vi "Do_ADAM_channel.vi"(4 "Scan Period":dbl format="%.2f", 5 "Previous Scan Value":dbl format="%.2f", 6 "Present scan array":dbl[](array[numeric]) format="%.2f", 7 "Value to Output":dbl format="%.2f", 8 "Ch Description":T1 {"Duty" format="%.0b"; "D" format="%#_5g"; "C" format="%#_5g"; "B" format="%#_5g"; "A" format="%#_5g"}, 9 "Ch names":string[](array[string])) -> (0 "Scan comment":string, 1 "Output":dbl format="%.3f")   [LabVIEW 2015]
uses:
  ADAM Client/Sub VIs/ADAM Controls/Ch_description_ADAM.ctl
  ADAM Client/Sub VIs/ADAM Controls/Module_type_ADAM.ctl
  ADAM Client/Sub VIs/ADAM Controls/Function_ADAM.ctl
  ADAM Client/Sub VIs/ADAM Controls/Channel_State.ctl
  ADAM Client/Sub VIs/ADAM Controls/Calib_type_ADAM.ctl
  ADAM Client/Sub VIs/ADAM Controls/Address.ctl
  ADAM Client/Sub VIs/ADAM Controls/Remember_value_mode.ctl
  ADAM Serial/Instrument drivers/Arduino/ctls_and_globals/Arduino tx msg cluster.ctl
  ADAM Client/Sub VIs/ADAM Controls/Search_mode.ctl
  Anemometry/Anemometry Sub Vis/Controls/In_Range.ctl
  <vilib>/Analysis/baseanly.llb/Mean (DBL).vi
  ADAM_Global.vi
  Anemometry/Anemometry Sub Vis/Globals/Gas_management_global.vi
  Anemometry/Anemometry Sub Vis/Globals/Constants_global.vi
  <vilib>/Analysis/NI_AALBase.lvlib
panel:
  in  "History Length":i32=150
  in  "K_Uni_chilled water":dbl=4.5
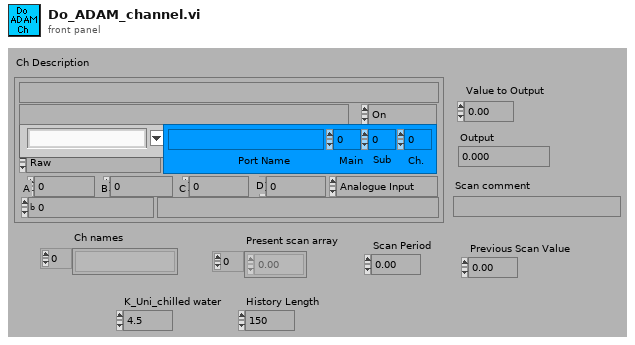
[diagram p1: front panel]
types:
  T1 = typedef "Ch_description_ADAM.ctl" = cluster{"Ch Name":string, "Type":T2, "Function":T3, "Ch State":T4, "Calibration type":T5, "A":dbl, "B":dbl, "C":dbl, "D":dbl, "Comments":string, "Address":T6, "String":string, "Duty":u16}
  T2 = typedef "Module_type_ADAM.ctl" = string
  T3 = typedef "Function_ADAM.ctl" = enum16{"Analogue Input", "Digital Input", "Event counter", "Event rate", "Analogue Output", "Digital Output", "Relay Output"}
  T4 = typedef "Channel_State.ctl" = enum16{"On", "Off", "Always On", "Always Off"}
  T5 = typedef "Calib_type_ADAM.ctl" = enum16{"Raw", "Bx + A", "Cx^2 + Bx + A", "Dx^3 + Cx^2 + Bx + A", "In Band", "Hi-Tec Q", "Hi-Tec M_dot", "Text"}
  T6 = typedef "Address.ctl" = cluster{"Main":i32, "Ch.":i32, "Sub":i32, "Port Name":string}
  T7 = typedef "Remember_value_mode.ctl" = enum16{"Read only", "Read and Write"}
  T8 = typedef "Search_mode.ctl" = enum16{"Between times", "All Times"}
  T9 = typedef "In_Range.ctl" = enum16{"%", "±", "% & ±"}
  T10 = typedef "Arduino tx msg cluster.ctl" = cluster{"dest":u8, "A/D/C/I":string, "R/W":string, "chan":u8, "val (float)":sgl}
  T11 = typedef "Client_State_Cluster.ctl" = cluster{"Client Name":string, "Traverse level State":T12, "People to Email":string[], "Next Contact Time":dbl}
  T12 = typedef "Traverse_Level_State.ctl" = enum16{"Running", "Complete"}
  T13 = cluster{"Centre Times":dbl[], "Output array":dbl[]}
  T14 = cluster{"Centre Times":dbl[], "Output array":dbl[]}[]
  T15 = typedef "Valco_valve_ph.ctl" = u16
  T16 = typedef "LVDateTimeRec.ctl" = cluster{"fractional second":dbl, "second":i32, "minute":i32, "hour":i32, "day of month":i32, "month":i32, "year":i32, "day of week":i32, "day of year":i32, "DST":i32}
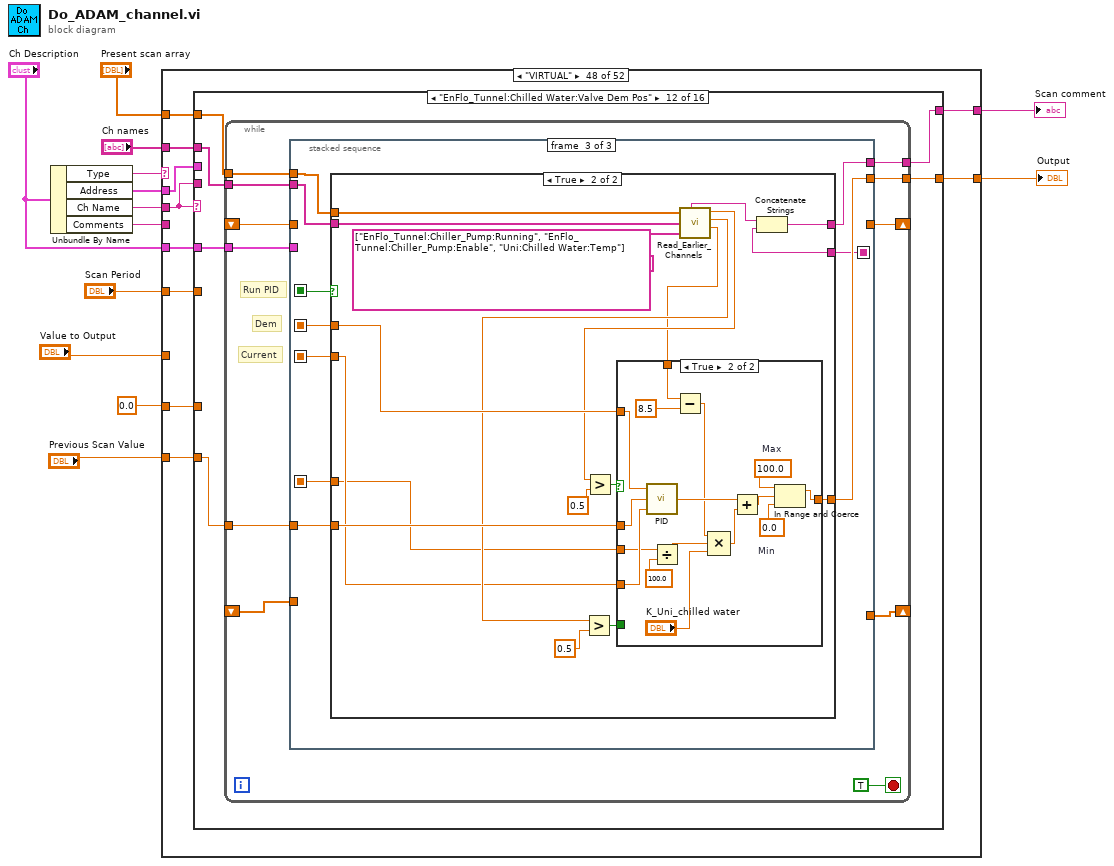
[diagram p0: block diagram]
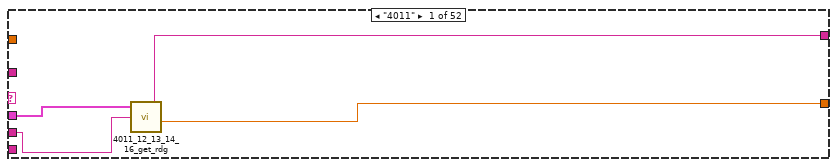
[diagram p2: hidden frame]
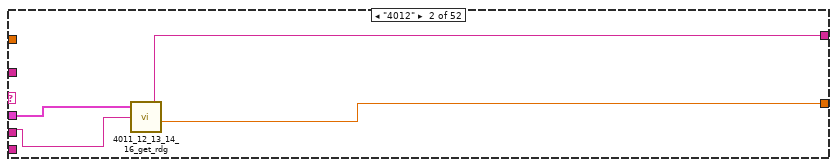
[diagram p3: hidden frame]
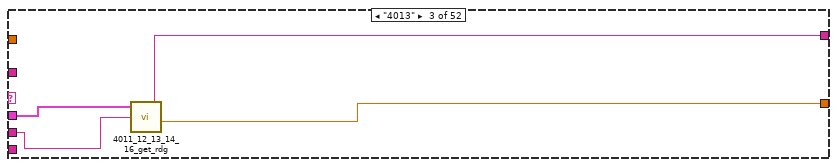
[diagram p4: hidden frame]
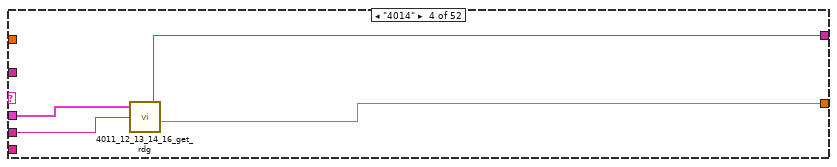
[diagram p5: hidden frame]
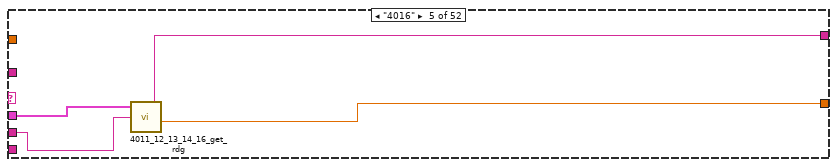
[diagram p6: hidden frame]
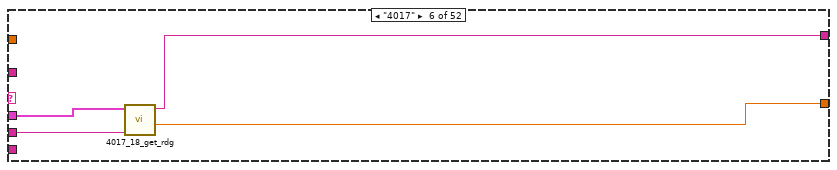
[diagram p7: hidden frame]
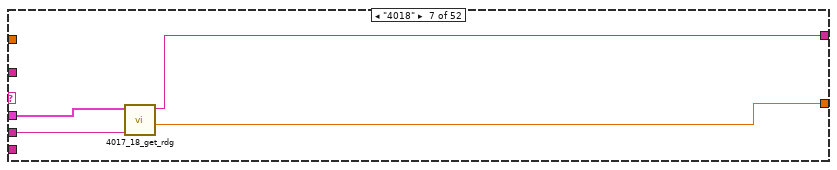
[diagram p8: hidden frame]
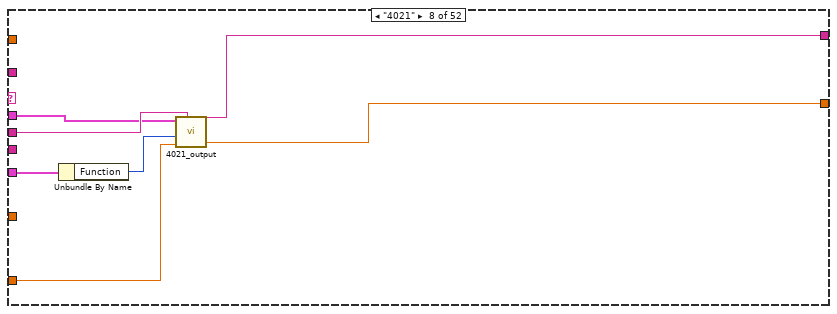
[diagram p9: hidden frame]
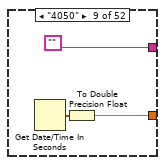
[diagram p10: hidden frame]
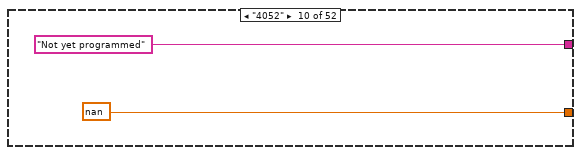
[diagram p11: hidden frame]
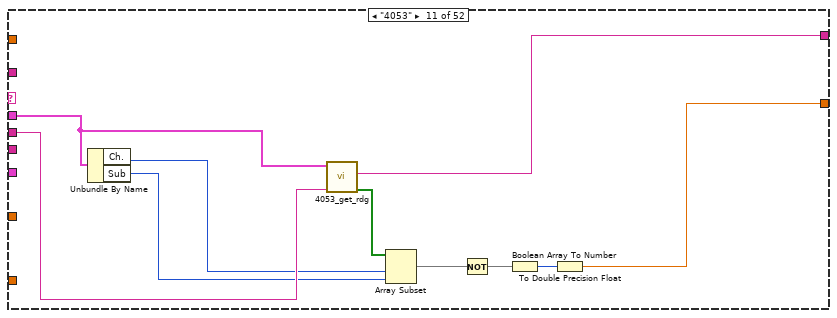
[diagram p12: hidden frame]
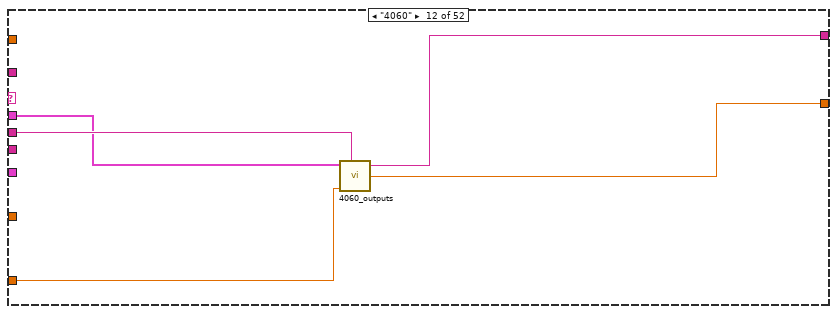
[diagram p13: hidden frame]
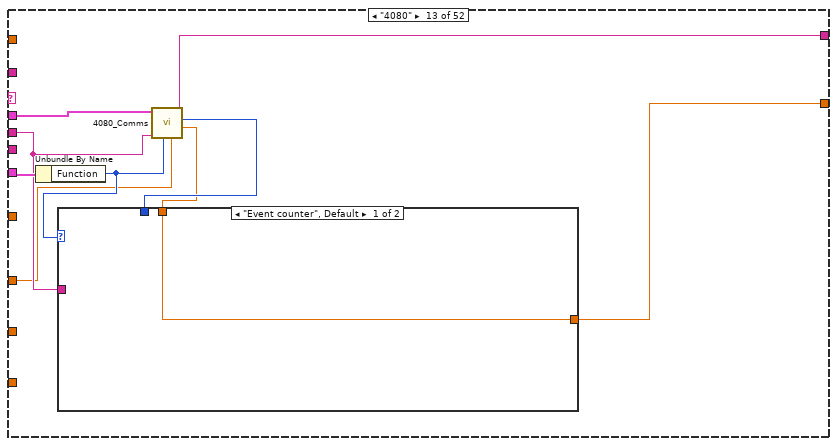
[diagram p14: hidden frame]
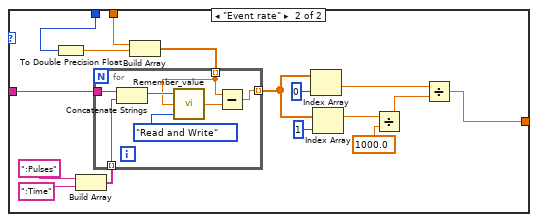
[diagram p15: hidden frame]
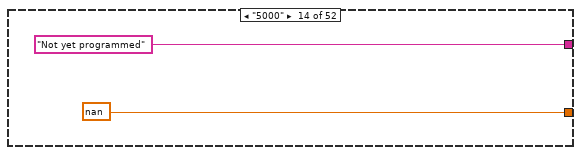
[diagram p16: hidden frame]
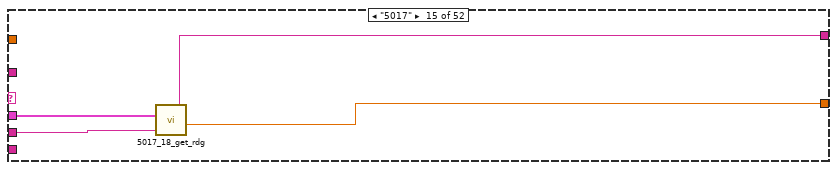
[diagram p17: hidden frame]
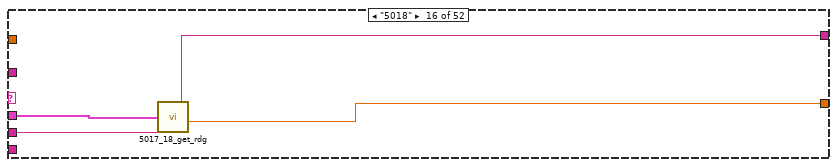
[diagram p18: hidden frame]
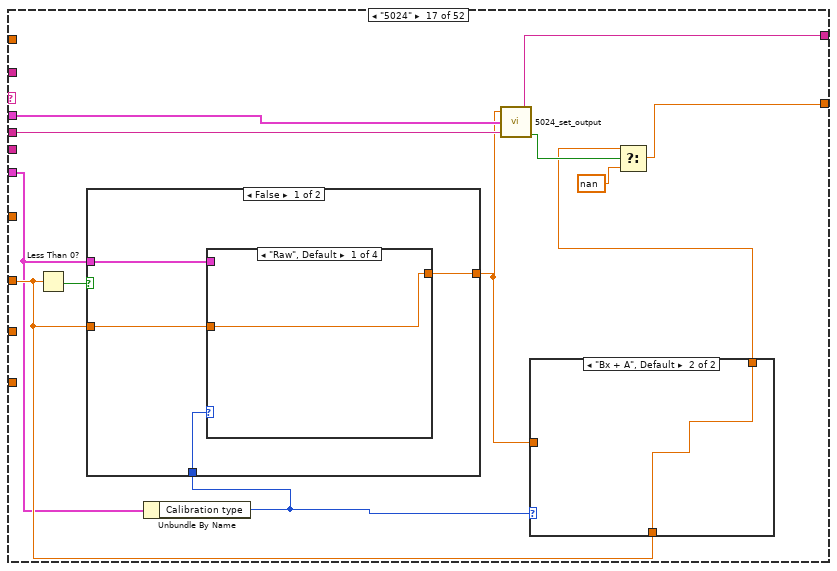
[diagram p19: hidden frame]
diagram:
  n1 = Unbundle By Name("Ch Description") -> ("Type"=w11:T2, "Address"=w10:T6, "Ch Name"=w2:string, "Comments"=w7:string)
  n2 = case shown="\"VIRTUAL\"" w11 {
    tunnel: [w16 w20 w24 w28 w32 w36 w40 w47 w50 nan w57 w66 w75 nan w105 w109 w119 w151 w159 w180 w202 w221 w236 w252 w281 w301 w389 w402 w404 w406 nan w514 w515 w518 w534 w546 0.0 ("Output") w555 w556 w560 w568 w599 w607 w690 w691 w697 w771 w819 w1340 nan w1371 w1397] -> w8
    tunnel: [w17 w21 w25 w29 w33 w37 w41 w48 "" "Not yet programmed" w62 w67 w77 "Not yet programmed" w106 w110 w122 w152 w158 w181 w203 w220 w239 w254 w276 w298 "" w403 "" w427 "Not yet programmed" w513 "" w519 w533 w547 "Warning; unmatched case in Do_ADAM_channel" ("Status note") w554 "" w561 w567 w598 w601 "Crazy time based random number!" w695 w699 w763 w818 w1341 "Not yet programmed" w1360 ""] -> w5
    tunnel: w10 -> [w14 w18 w22 w26 w30 w34 w38 w42 _ _ w54 w65 w69 _ w107 w111 w123 w153 w157 w182 w204 w235 w251 w267 w292 _ _ w401 _ _ _ w511 _ w517 w536 w549 _ w552 _ _ _ _ _ _ w693 w701 w768 w810 w1346 _ _ w1406]
    tunnel: "Ch Description" -> [_ _ _ _ _ _ _ w46 _ _ _ _ w76 _ _ _ w112 _ w156 w179 w201 _ _ _ _ w305 _ _ _ w432 _ _ _ _ _ _ _ _ w557 w562 w573 w600 w605 _ _ w700 _ w812 _ _ _ _]
    tunnel: w2 -> [w15 w19 w23 w27 w31 w35 w39 w43 _ _ w63 w68 w72 _ w104 w108 w118 w150 w154 w176 w198 _ _ _ _ _ w385 _ _ _ _ w512 _ _ w535 w548 _ w553 _ _ _ _ _ _ w694 w698 w764 w815 w1345 _ w1367 _]
    tunnel: "Ch names" -> [_ _ _ _ _ _ _ _ _ _ _ _ _ _ _ _ _ _ _ _ _ _ _ _ _ w310 _ _ _ w431 _ _ _ _ _ _ _ _ _ w563 w574 _ w613 _ _ _ _ w817 _ _ _ _]
    tunnel: "Present scan array" -> [_ _ _ _ _ _ _ _ _ _ _ _ _ _ _ _ _ _ _ _ _ _ _ _ _ w309 _ _ _ w429 _ _ _ _ _ _ _ _ _ w564 w571 _ w612 _ _ _ _ w816 _ _ _ _]
    tunnel: w7 -> [_ _ _ _ _ _ _ _ _ _ _ _ _ _ _ _ _ _ _ _ _ _ _ _ _ w308 _ _ _ w433 _ _ _ _ _ _ _ _ _ _ w566 _ w611 _ _ _ _ _ _ _ _ _]
    tunnel: "Value to Output" -> [_ _ _ _ _ _ _ w44 _ _ _ w64 w70 _ _ _ w114 _ w155 w177 w199 _ w237 w253 _ _ _ _ _ _ _ _ _ _ w532 _ _ _ _ _ w572 _ _ _ _ w696 w772 _ _ _ _ w1401]
    tunnel: "Scan Period" -> [_ _ _ _ _ _ _ _ _ _ _ _ _ _ _ _ _ _ _ _ _ _ _ _ _ w300 _ _ _ _ _ _ _ _ _ _ _ _ _ _ w569 _ w606 _ _ _ _ w814 _ _ _ _]
    tunnel: "Previous Scan Value" -> [_ _ _ _ _ _ _ _ _ _ _ _ _ _ _ _ _ _ _ _ _ w223 _ _ w268 _ _ _ w404 w407 _ _ w515 _ _ _ _ _ _ _ w570 _ _ _ _ _ _ w813 _ _ _ _]
    tunnel: 0.0 -> [_ _ _ _ _ _ _ _ _ _ _ _ _ _ _ _ _ _ _ _ _ _ _ _ _ _ _ _ _ _ _ _ _ _ _ _ _ _ _ _ _ _ _ _ _ _ _ w811 _ _ _ _]
    frame "4011" {
      n3 = call "4011_12_13_14_16_get_rdg.vi"("Address"=w14, "Channel Name"=w15) -> ("Comment"=w17:string, "Reading"=w16:dbl)  [unwired: 1 in, 2 out]
    }
    frame "4012" {
      n4 = call "4011_12_13_14_16_get_rdg.vi"("Address"=w18, "Channel Name"=w19) -> ("Comment"=w21:string, "Reading"=w20:dbl)  [unwired: 1 in, 2 out]
    }
    frame "4013" {
      n5 = call "4011_12_13_14_16_get_rdg.vi"("Address"=w22, "Channel Name"=w23) -> ("Comment"=w25:string, "Reading"=w24:dbl)  [unwired: 1 in, 2 out]
    }
    frame "4014" {
      n6 = call "4011_12_13_14_16_get_rdg.vi"("Address"=w26, "Channel Name"=w27) -> ("Comment"=w29:string, "Reading"=w28:dbl)  [unwired: 1 in, 2 out]
    }
    frame "4016" {
      n7 = call "4011_12_13_14_16_get_rdg.vi"("Address"=w30, "Channel Name"=w31) -> ("Comment"=w33:string, "Reading"=w32:dbl)  [unwired: 1 in, 2 out]
    }
    frame "4017" {
      n8 = call "4017_18_get_rdg.vi"("Channel Name"=w35, "Address"=w34) -> ("Reading"=w36:dbl, "Comment"=w37:string)  [unwired: 2 in, 2 out]
    }
    frame "4018" {
      n9 = call "4017_18_get_rdg.vi"("Channel Name"=w39, "Address"=w38) -> ("Reading"=w40:dbl, "Comment"=w41:string)  [unwired: 2 in, 2 out]
    }
    frame "4021" {
      n10 = Unbundle By Name(w46) -> ("Function"=w45:T3)
      n11 = call "4021_output.vi"("Address"=w42, "Function"=w45, "Set to:"=w44, "Channel Name"=w43) -> ("Comment"=w48:string, "Reading"=w47:dbl)  [unwired: 1 in, 1 out]
    }
    frame "4050" {
      n12 = Get Date/Time In Seconds() -> (seconds since 1Jan1904=w49:timestamp)
      n13 = To Double Precision Float(number=w49) -> (double precision float=w50:dbl)
    }
    frame "4052" {
    }
    frame "4053" {
      n14 = Unbundle By Name(w54) -> ("Ch."=w55:i32, "Sub"=w61:i32)
      n15 = call "4053_get_rdg.vi"("Channel Name"=w63, "Address"=w54) -> ("Boolean array"=w60:bool[], "Comment"=w62:string)  [unwired: 2 in, 2 out]
      n16 = Array Subset(array=w60, index=w55, length=w61) -> (w59:bool[])
      n17 = Not(x=w59) -> (.not. x?=w56:bool[])
      n18 = Boolean Array To Number(Boolean array=w56) -> (number=w58:u32)
      n19 = To Double Precision Float(number=w58) -> (double precision float=w57:dbl)
    }
    frame "4060" {
      n20 = call "4060_outputs.vi"("Address"=w65, "Value to Output"=w64, "Channel Name"=w68) -> ("Comment"=w67:string, "Reading"=w66:dbl)  [unwired: 2 in, 1 out]
    }
    frame "4080" {
      n21 = Unbundle By Name(w76) -> ("Function"=w71:T3)
      n22 = call "4080_Comms.vi"("Value to display"=w70, "Function"=w71, "Channel Name"=w72, "Address"=w69) -> ("Reading"=w73:dbl, "millisecond timer value"=w74:u32, "Comment"=w77:string)  [unwired: 2 in, 1 out]
      n23 = case shown="\"Event counter\", Default" w71 {
        tunnel: w72 -> [_ w94]
        tunnel: w74 -> [_ w87]
        tunnel: [w78 w79] -> w75
        tunnel: w73 -> [w78 w88]
        frame "Event counter", Default {
        }
        frame "Event rate" {
          n24 = To Double Precision Float(number=w87) -> (double precision float=w86:dbl)
          n25 = Build Array(":Pulses", ":Time") -> (w89:string[])
          n26 = Build Array(w88, w86) -> (w85:dbl[])
          n27 = for {
            tunnel: w94 -> [w98]
            tunnel: [w99] -> w82 mode=indexing
            tunnel: w89 -> [w96] mode=indexing
            tunnel: w85 -> [w95] mode=indexing
            n28 = Concatenate Strings(w98, w96) -> (w97:string)
            n29 = call "Remember_value.vi"("Mode"=Remember_value_mode."Read and Write", "Input Value"=w95, "Ch name"=w97) -> ("Output Value"=w100:dbl)
            n30 = Subtract(x=w95, y=w100) -> (x-y=w99:dbl)
          }
          n31 = Index Array(array=w82, index=0) -> (element=w80:dbl)
          n32 = Index Array(array=w82, index=1) -> (element=w81:dbl)
          n33 = Divide(x=w81, y=1000.0) -> (x/y=w92:dbl)
          n34 = Divide(x=w80, y=w92) -> (x/y=w79:dbl)
        }
      }
    }
    frame "5000" {
    }
    frame "5017" {
      n35 = call "5017_18_get_rdg.vi"("Address (all reqd.)"=w107, "Channel Name"=w104) -> ("Comment"=w106:string, "Reading"=w105:dbl)  [unwired: 3 out]
    }
    frame "5018" {
      n36 = call "5017_18_get_rdg.vi"("Address (all reqd.)"=w111, "Channel Name"=w108) -> ("Comment"=w110:string, "Reading"=w109:dbl)  [unwired: 3 out]
    }
    frame "5024" {
      n37 = Less Than 0?(x=w114) -> (x < 0?=w117:bool)
      n38 = Unbundle By Name(w112) -> ("Calibration type"=w113:T5)
      n39 = case shown="False" w117 {
        tunnel: [w129 0.0 ("t")] -> w115
        tunnel: w114 -> [w127 _]
        tunnel: w113 -> [w128 _]
        tunnel: w112 -> [w126 _]
        frame False {
          n40 = case shown="\"Raw\", Default" w128 {
            tunnel: w127 -> [w130 w133 w139 w145]
            tunnel: w126 -> [_ w136 w142 w148]
            tunnel: [w130 w131 w137 w143] -> w129
            frame "Raw", Default {
            }
            frame "Bx + A" {
              n41 = Unbundle By Name(w136) -> ("A"=w135:dbl)
              n42 = Equal?(x=w135, y=w133) -> (x = y?=w134:bool)
              n43 = Select(t=0.0, s=w134, f=w133) -> (s? t:f=w131:dbl)
            }
            frame "Cx^2 + Bx + A" {
              n44 = Unbundle By Name(w142) -> ("A"=w141:dbl)
              n45 = Equal?(x=w141, y=w139) -> (x = y?=w140:bool)
              n46 = Select(t=0.0, s=w140, f=w139) -> (s? t:f=w137:dbl)
            }
            frame "Dx^3 + Cx^2 + Bx + A" {
              n47 = Unbundle By Name(w148) -> ("A"=w147:dbl)
              n48 = Equal?(x=w147, y=w145) -> (x = y?=w146:bool)
              n49 = Select(t=0.0, s=w146, f=w145) -> (s? t:f=w143:dbl)
            }
          }
        }
        frame True {
        }
      }
      n50 = call "5024_set_output.vi"("Set to:"=w115, "Address (all reqd.)"=w123, "Channel Name"=w118) -> ("Comment"=w122:string, "Good Reply"=w120:bool)  [unwired: 2 out]
      n51 = case shown="\"Bx + A\", Default" w113 {
        tunnel: [w124 w125] -> w116
        tunnel: w115 -> [w124 _]
        tunnel: w114 -> [_ w125]
        frame "Raw" {
        }
        frame "Bx + A", Default {
        }
      }
      n52 = Select(t=w116, s=w120, f=nan) -> (s? t:f=w119:dbl)
    }
    frame "5051" {
      n53 = call "5051_56_get_inputs.vi"("Address (Main, Sub reqd.)"=w153, "Channel Name"=w150) -> ("Comment"=w152:string, "Single output"=w151:dbl)  [unwired: 3 out]
    }
    frame "5056" {
      n54 = Unbundle By Name(w156) -> ("Function"=w160:T3)
      n55 = case shown="\"Digital Input\"" w160 {
        tunnel: w157 -> [_ w166 w175]
        tunnel: ["This function is not available" w167 w173] -> w158
        tunnel: [nan ("A") w164 w170] -> w159
        tunnel: w155 -> [_ _ w169]
        tunnel: w154 -> [_ w163 w168]
        frame "Analogue Input", Default {
        }
        frame "Digital Input" {
          # "Readback value"
          n56 = call "5060_check_outputs.vi"("Address (Main, Sub reqd.)"=w166, "Channel Name"=w163) -> ("Comment"=w167:string, "Single Channel"=w165:i16)  [unwired: 3 out]
          n57 = To Double Precision Float(number=w165) -> (double precision float=w164:dbl)
        }
        frame "Relay Output" {
          # "Sets single o/p channel"
          n58 = Greater Than 0?(x=w169) -> (x > 0?=w174:bool)
          n59 = call "5056_60_set_single_output.vi"("Channel Name"=w168, "Address (all reqd.)"=w175, "Set state:"=w174) -> ("Comment"=w173:string, "Good Reply"=w172:bool)  [unwired: 2 out]
          n60 = Select(t=w169, s=w172, f=nan) -> (s? t:f=w170:dbl)
        }
      }
    }
    frame "5060" {
      n61 = Unbundle By Name(w179) -> ("Function"=w178:T3)
      n62 = case shown="\"Relay Output\"" w178 {
        tunnel: w182 -> [_ w188 w197]
        tunnel: ["This function is not available" w189 w195] -> w181
        tunnel: [nan ("A") w186 w192] -> w180
        tunnel: w177 -> [_ _ w191]
        tunnel: w176 -> [_ w185 w190]
        frame "Analogue Input", Default {
        }
        frame "Digital Input" {
          # "Readback value"
          n63 = call "5060_check_outputs.vi"("Address (Main, Sub reqd.)"=w188, "Channel Name"=w185) -> ("Comment"=w189:string, "Single Channel"=w187:i16)  [unwired: 3 out]
          n64 = To Double Precision Float(number=w187) -> (double precision float=w186:dbl)
        }
        frame "Relay Output" {
          # "Sets single o/p channel"
          n65 = Greater Than 0?(x=w191) -> (x > 0?=w196:bool)
          n66 = call "5056_60_set_single_output.vi"("Channel Name"=w190, "Address (all reqd.)"=w197, "Set state:"=w196) -> ("Comment"=w195:string, "Good Reply"=w194:bool)  [unwired: 2 out]
          n67 = Select(t=w191, s=w194, f=nan) -> (s? t:f=w192:dbl)
        }
      }
    }
    frame "6060" {
      n68 = Unbundle By Name(w201) -> ("Function"=w200:T3)
      n69 = case shown="\"Digital Input\"" w200 {
        tunnel: w204 -> [_ w210 w219]
        tunnel: ["This function is not available" w211 w217] -> w203
        tunnel: [nan ("A") w208 w214] -> w202
        tunnel: w199 -> [_ _ w213]
        tunnel: w198 -> [_ w207 w212]
        frame "Analogue Input", Default {
        }
        frame "Digital Input" {
          n70 = call "6060_read_all_I-O.vi"("Address (Main, Sub reqd.)"=w210, "Channel Name"=w207) -> ("Comment"=w211:string, "Single Input Channel"=w209:i16)  [unwired: 3 out]
          n71 = To Double Precision Float(number=w209) -> (double precision float=w208:dbl)
        }
        frame "Relay Output" {
          # "Sets single o/p channel"
          n72 = Greater Than 0?(x=w213) -> (x > 0?=w218:bool)
          n73 = call "6060_set_single_output.vi"("Channel Name"=w212, "Address (Main, Ch requd.)"=w219, "Set state:"=w218) -> ("Comment"=w217:string, "Good Reply"=w216:bool)  [unwired: 2 out]
          n74 = Select(t=w213, s=w216, f=nan) -> (s? t:f=w214:dbl)
        }
      }
    }
    frame "Arduino A_in" {
      w229 = T10 {"dest"=1, "A/D/C/I"="A", "R/W"="R", "chan"=1, "val (float)"=0.0}  # Tx msg cluster
      # "Analogue read case"
      n75 = Unbundle By Name(w235) -> ("Port Name"=w226:string, "Main"=w227:i32, "Ch."=w228:i32)
      n76 = To Unsigned Byte Integer(number=w227) -> (unsigned 8bit integer=w234:u8)
      n77 = To Unsigned Byte Integer(number=w228) -> (unsigned 8bit integer=w232:u8)
      n78 = Bundle By Name(cluster=w229, "dest"=w234, "A/D/C/I"="A" ("A/D"), "R/W"="R", "chan"=w232, "val (float)"=sgl 0.0) -> (w225:T10)
      n79 = call "Arduino generic wrapper.vi"("Tx msg cluster"=w225, "Port name"=w226) -> ("Scan comment"=w220:string, "Output"=w222:dbl)
      n80 = Empty String/Path?(string/path=w220) -> (empty?=w224:bool)
      n81 = Select(t=w222, s=w224, f=w223) -> (s? t:f=w221:dbl)
    }
    frame "Arduino A_out" {
      w246 = T10 {"dest"=1, "A/D/C/I"="A", "R/W"="R", "chan"=1, "val (float)"=0.0}  # Tx msg cluster
      # "Analogue write case"
      n82 = Unbundle By Name(w251) -> ("Port Name"=w243:string, "Main"=w244:i32, "Ch."=w245:i32)
      n83 = To Unsigned Byte Integer(number=w244) -> (unsigned 8bit integer=w250:u8)
      n84 = To Unsigned Byte Integer(number=w245) -> (unsigned 8bit integer=w249:u8)
      n85 = To Single Precision Float(number=w237) -> (single precision float=w241:sgl)
      n86 = Bundle By Name(cluster=w246, "dest"=w250, "A/D/C/I"="A" ("A/D"), "R/W"="W", "chan"=w249, "val (float)"=w241) -> (w242:T10)
      n87 = call "Arduino generic wrapper.vi"("Tx msg cluster"=w242, "Port name"=w243) -> ("Scan comment"=w239:string)  [unwired: 1 out]
      n88 = Empty String/Path?(string/path=w239) -> (empty?=w238:bool)
      n89 = Select(t=w237, s=w238, f=nan ("Reading")) -> (s? t:f=w236:dbl)
    }
    frame "Arduino D_out" {
      w262 = T10 {"dest"=1, "A/D/C/I"="A", "R/W"="R", "chan"=1, "val (float)"=0.0}  # Tx msg cluster
      # "Digital write case"
      n90 = Unbundle By Name(w267) -> ("Port Name"=w259:string, "Main"=w260:i32, "Ch."=w261:i32)
      n91 = To Unsigned Byte Integer(number=w260) -> (unsigned 8bit integer=w266:u8)
      n92 = To Unsigned Byte Integer(number=w261) -> (unsigned 8bit integer=w265:u8)
      n93 = To Single Precision Float(number=w253) -> (single precision float=w257:sgl)
      n94 = Bundle By Name(cluster=w262, "dest"=w266, "A/D/C/I"="D" ("A/D"), "R/W"="W", "chan"=w265, "val (float)"=w257) -> (w258:T10)
      n95 = call "Arduino generic wrapper.vi"("Tx msg cluster"=w258, "Port name"=w259) -> ("Scan comment"=w254:string)  [unwired: 1 out]
      n96 = Empty String/Path?(string/path=w254) -> (empty?=w255:bool)
      n97 = Select(t=w253, s=w255, f=nan ("Reading")) -> (s? t:f=w252:dbl)
    }
    frame "Arduino Thermistor" {
      w286 = T10 {"dest"=1, "A/D/C/I"="A", "R/W"="R", "chan"=1, "val (float)"=0.0}  # Tx msg cluster
      # "Thermistor read case"
      # "values not expected in 'normal' operating conditions"
      n98 = Unbundle By Name(w292) -> ("Port Name"=w283:string, "Main"=w284:i32, "Ch."=w285:i32)
      n99 = To Unsigned Byte Integer(number=w284) -> (unsigned 8bit integer=w291:u8)
      n100 = To Unsigned Byte Integer(number=w285) -> (unsigned 8bit integer=w289:u8)
      n101 = Bundle By Name(cluster=w286, "dest"=w291, "A/D/C/I"="A" ("A/D"), "R/W"="R", "chan"=w289, "val (float)"=sgl 0.0) -> (w282:T10)
      n102 = call "Arduino generic wrapper.vi"("Tx msg cluster"=w282, "Port name"=w283) -> ("Scan comment"=w272:string, "Output"=w270:dbl)
      n103 = Empty String/Path?(string/path=w272) -> (empty?=w271:bool)
      n104 = Select(t=w270, s=w271, f=w268) -> (s? t:f=w269:dbl)
      n105 = Less?(x=w270, y=-40.0) -> (x < y?=w273:bool)
      n106 = Greater?(x=w270, y=140.0) -> (0:w274:bool)
      n107 = case shown="False" w273 {
        tunnel: [w294 "Faulty thermistor open-circuit;"] -> w275
        tunnel: w274 -> [w293 _]
        frame False {
          n108 = case shown="True" w293 {
            tunnel: ["" "Faulty thermistor short-circuit;"] -> w294
            frame False {
            }
            frame True {
            }
          }
        }
        frame True {
        }
      }
      n109 = Or(x=w273, y=w274) -> (x .or. y?=w278:bool)
      n110 = Select(t=nan ("f"), s=w278, f=w269) -> (s? t:f=w281:dbl)
      n111 = Concatenate Strings(w272, w275) -> (w276:string)
    }
    frame "Average" {
      # "The Channel names to average must appear in the comments field separated by semi colons"
      n112 = call "Get_array_values_fr_String.vi"("String Value"=w308) -> ("String array"=w307:string[])  [unwired: 1 out]
      n113 = Equal To 0?(x=w300) -> (x = 0?=w299:bool)
      n114 = global read "ADAM_Global.vi" "Active Ch names"() -> (w306:string[])
      n115 = case shown="False" w299 {
        tunnel: w305 -> [w314 _]
        tunnel: [w312 TRUE] -> w304
        tunnel: [w311 2.0 ("A")] -> w303
        frame False {
          n116 = Unbundle By Name(w314) -> ("D"=w311:dbl)
          n117 = Less?(x=w311, y=2.0) -> (x < y?=w312:bool)
        }
        frame True {
        }
      }
      n118 = case shown="True" w304 {
        tunnel: w310 -> [_ w349]
        tunnel: w309 -> [_ w348]
        tunnel: w307 -> [w319 w347]
        tunnel: [w317 w345] -> w298
        tunnel: w306 -> [_ w344]
        tunnel: [w320 w343] -> w302
        tunnel: w303 -> [w321 _]
        frame False {
          w328 = FALSE  # All Active Channels
          n119 = Get Date/Time In Seconds() -> (seconds since 1Jan1904=w331:timestamp)
          n120 = To Double Precision Float(number=w331) -> (double precision float=w329:dbl)
          n121 = Subtract(x=w329, y=w321) -> (x-y=w330:dbl)
          n122 = call "Get_ADAM_averages_server.vi"("No of averages"=1, "All Active Channels"=w328, "End time"=w329, "Start time"=w330, "Clients time"=w329, "ADAM Ch Names"=w319) -> ("DBL values"=w326:dbl[][])  [unwired: 4 out]
          n123 = Index Array(array=w326, index (row)=0) -> (element=w323:dbl[])  [unwired: 1 in]
          n124 = Array Subset(array=w323, index=1) -> (w322:dbl[])  [unwired: 1 in]
          n125 = for {
            tunnel: w322 -> [w337] mode=indexing
            tunnel: [w337] -> w320 mode=indexing if=w335
            tunnel: w319 -> [w334] mode=indexing
            shift-right: [w332] -> w317
            shift-left: "" -> [w333]
            n126 = Not A Number/Path/Refnum?(number/path/refnum=w337) -> (NaN/Path/Refnum?=w336:bool)
            n127 = Not(x=w336) -> (.not. x?=w335:bool)
            n128 = case shown="False" w335 {
              tunnel: w334 -> [w340 _]
              tunnel: w333 -> [w339 w342]
              tunnel: [w338 w342] -> w332
              frame False {
                n129 = Format Into String(format string="Channel \"%s\" is not currently active.\n", initial string=w339, w340) -> (resulting string=w338:string)  [unwired: 1 in, 1 out]
              }
              frame True {
              }
            }
          }
        }
        frame True {
          n130 = for {
            tunnel: w349 -> [w362]
            tunnel: w348 -> [w361]
            tunnel: w347 -> [w358] mode=indexing
            shift-right: [w359] -> w345
            shift-left: "" -> [w360]
            tunnel: [w352] -> w343 mode=indexing if=w350
            tunnel: w344 -> [w353]
            n131 = call "Read_value_of_earlier_Ch.vi"("Desired Ch to Read"=w358, "Ch names"=w362, "Present scan array"=w361) -> ("Value"=w356:dbl, "Scan comment"=w355:string)  [unwired: 1 in]
            n132 = Not A Number/Path/Refnum?(number/path/refnum=w356) -> (NaN/Path/Refnum?=w357:bool)
            n133 = case shown="False" w357 {
              tunnel: w358 -> [w365 _]
              tunnel: [w368 w378] -> w352
              tunnel: w356 -> [w367 w378]
              tunnel: [w370 w377] -> w354
              tunnel: w355 -> [w369 w377]
              tunnel: w353 -> [w366 _]
              frame False {
                n134 = Search 1D Array(1D array=w366, element=w365) -> (index of element=w363:i32)  [unwired: 1 in]
                n135 = Greater Or Equal To 0?(x=w363) -> (x >= 0?=w364:bool)
                n136 = case shown="False" w364 {
                  tunnel: w365 -> [w374 _]
                  tunnel: [w373 w376] -> w370
                  tunnel: w369 -> [_ w376]
                  tunnel: [nan w375] -> w368
                  tunnel: w367 -> [_ w375]
                  frame False {
                    n137 = Format Into String(format string="Channel \"%s\" is not currently active.\n", w374) -> (resulting string=w373:string)  [unwired: 2 in, 1 out]
                  }
                  frame True {
                  }
                }
              }
              frame True {
              }
            }
            n138 = Concatenate Strings(w360, w354) -> (w359:string)
            n139 = Not A Number/Path/Refnum?(number/path/refnum=w352) -> (NaN/Path/Refnum?=w351:bool)
            n140 = Not(x=w351) -> (.not. x?=w350:bool)
          }
        }
      }
      n141 = call-poly <vilib>:"Mean.vi"("X"=w302) -> ("mean"=w301:dbl)  [unwired: 1 out]
    }
    frame "Client Info" {
      n142 = global read "ADAM_Global.vi" "Client State Array"() -> (w391:T11[])
      n143 = call "Split_Ch_name.vi"("Ch name"=w385) -> ("Top level"=w383:string, "Low level"=w381:string)  [unwired: 1 out]
      n144 = Equal?(x="Status" ("Substring"), y=w383) -> (x = y?=w382:bool)
      n145 = Select(t=w381, s=w382, f="") -> (s? t:f=w379:string)
      n146 = for {
        tunnel: w391 -> [w400] mode=indexing
        tunnel: [w399] -> w392 mode=indexing
        n147 = Unbundle By Name(w400) -> ("Client Name"=w399:string)
      }
      n148 = Search 1D Array(1D array=w392, element=w379) -> (index of element=w387:i32)  [unwired: 1 out]
      n149 = Less Than 0?(x=w387) -> (x < 0?=w386:bool)
      n150 = Index Array(array=w391, index=w387) -> (element=w390:T11)
      n151 = case shown="False" w386 {
        tunnel: w390 -> [w395 _]
        tunnel: w379 -> [w394 w397]
        tunnel: [w393 w396] -> w389
        frame False {
          n152 = call "Get_Client_Status_string.vi"("Client State Cluster"=w395, "Client Name"=w394) -> ("Code Value"=w393:dbl)  [unwired: 1 in]
        }
        frame True {
          w396 = 7.0 ("Code Value")
          n153 = call "Remember_value.vi"("Mode"=Remember_value_mode."Read and Write", "Input Value"=w396, "Ch name"=w397) -> ()  [unwired: 1 out]
        }
      }
    }
    frame "ClimatronicsUDP" {
      n154 = call "ClimatronicsUDP_get_rdg.vi"("Address"=w401) -> ("Output"=w402:dbl, "Status note"=w403:string)  [unwired: 5 in]
    }
    frame "Coded" {
    }
    frame "Comparator" {
      # "A Warn if above this value\nB Warn if below this value\nC  Hysteresis margin\nD is the averaging time in minutes\nComments   is Channel name to check"
      n155 = Unbundle By Name(w432) -> ("D"=w415:dbl)
      n156 = Match Pattern(string=w433, regular expression=":::" ("String to match")) -> (before substring=w430:string)  [unwired: 4 out]
      n157 = call "Read_value_of_earlier_Ch.vi"("Desired Ch to Read"=w430, "Ch names"=w431, "Present scan array"=w429) -> ("Value"=w414:dbl, "Scan comment"=w428:string)  [unwired: 1 in]
      n158 = Equal?(x=w407, y=1.0) -> (x = y?=w423:bool)
      n159 = Unbundle By Name(w432) -> ("A"=w426:dbl, "B"=w425:dbl, "C"=w424:dbl)
      n160 = Equal To 0?(x=w415) -> (x = 0?=w413:bool)
      n161 = case shown="True" w423 {
        tunnel: [w439 w444] -> w421
        tunnel: w426 -> [w439 w443]
        tunnel: w425 -> [w438 w442]
        tunnel: [w438 w440] -> w422
        tunnel: w424 -> [_ w441]
        frame False {
        }
        frame True {
          n162 = Subtract(x=w443, y=w441) -> (x-y=w444:dbl)
          n163 = Add(x=w442, y=w441) -> (x+y=w440:dbl)
        }
      }
      n164 = case shown="False" w413 {
        tunnel: [w449 w452] -> w436
        tunnel: w430 -> [w451 _]
        tunnel: [w447 w453] -> w412
        tunnel: w415 -> [w445 _]
        tunnel: w414 -> [_ w453]
        tunnel: w428 -> [w449 w452]
        frame False {
          n165 = Build Array(w451) -> (w446:string[])
          n166 = call "Get_Channel_averages.vi"("Desired Ch Names"=w446, "Averaging time (mins)"=w445) -> ("number"=w448:dbl[])  [unwired: 1 in, 2 out]
          n167 = Index Array(array=w448, index=0) -> (element=w447:dbl)
        }
        frame True {
        }
      }
      n168 = Not(x=w423) -> (.not. x?=w416:bool)
      n169 = In Range and Coerce(upper limit=w421, x=w412, lower limit=w422) -> (In Range?=w417:bool)  [unwired: 1 out]
      n170 = Greater?(x=w412, y=w421) -> (0:w420:bool)
      n171 = Not A Number/Path/Refnum?(number/path/refnum=w412) -> (NaN/Path/Refnum?=w409:bool)
      n172 = Equal?(x=w417, y=w416) -> (x = y?=w411:bool)
      n173 = Or(x=w411, y=w409) -> (x .or. y?=w410:bool)
      n174 = case shown="False" w410 {
        tunnel: w430 -> [w460 _]
        tunnel: w421 -> [w459 _]
        tunnel: w432 -> [w458 _]
        tunnel: w422 -> [w457 _]
        tunnel: w417 -> [w456 _]
        tunnel: w412 -> [w455 _]
        tunnel: w420 -> [w454 _]
        frame False {
          n175 = stacked-sequence {
            seq-local: [w466 _ _ _ _] -> [_ _ _ w507 _]
            seq-local: [_ w486 _ _ _] -> [_ _ _ w504 _]
            seq-local: [w464 _ _ _ _] -> [_ _ _ w500 _]
            tunnel: w460 -> [w468 w494 _ w506 _]
            tunnel: w459 -> [w467 _ _ _ _]
            tunnel: w458 -> [_ _ w499 w508 _]
            tunnel: w457 -> [w465 _ _ _ _]
            tunnel: w456 -> [w463 _ _ _ _]
            tunnel: w455 -> [w462 _ _ _ _]
            tunnel: w454 -> [w461 _ _ _ _]
            frame #0 {
              n176 = case shown="True" w463 {
                tunnel: w468 -> [w473 w484]
                tunnel: w467 -> [_ w477]
                tunnel: [w471 w483] -> w466
                tunnel: w465 -> [_ w476]
                tunnel: ["OK " ""] -> w464
                tunnel: w462 -> [w469 _]
                tunnel: w461 -> [_ w474]
                frame True {
                  n177 = Format Into String(format string="The channel named %s is now  %.3f" ("Format String"), w473, w469) -> (resulting string=w471:string)  [unwired: 2 in, 1 out]
                }
                frame False {
                  n178 = Select(t=w477, s=w474, f=w476) -> (s? t:f=w475:dbl)
                  n179 = Select(t="greater", s=w474, f="less") -> (s? t:f=w479:string)
                  n180 = Format Into String(format string="%s is %s than %.3f" ("Format String"), w484, w479, w475) -> (resulting string=w483:string)  [unwired: 2 in, 1 out]
                }
              }
            }
            frame #1 {
              n181 = Build Array(w494) -> (w493:string[])
              n182 = call "Channel_Names_and_indicies.vi"("All Active Channels"=FALSE, "Desired Ch Names"=w493) -> ("Indicies"=w491:i32[])  [unwired: 1 out]
              n183 = call "Specified_Channels_server.vi"("Mode"=Search_mode."All Times", "Requested channels"=w491) -> ("Output array"=w489:dbl[][], "Centre Times"=w485:dbl[])  [unwired: 3 in, 3 out]
              n184 = Index Array(array=w489, index (row)=0) -> (element=w487:dbl[])  [unwired: 1 in]
              n185 = Bundle("Centre Times"=w485, "Output array"=w487) -> (w490:T13)  [unwired: 1 out]
              n186 = Build Array(w490) -> (w486:T14)
            }
            frame #2 {
              w497 = TRUE  # Contact All clients?
              n187 = Unbundle By Name(w499) -> ("String"=w498:string)
              n188 = call "Get_array_values_fr_String.vi"("String Value"=w498) -> ("String array"=w496:string[])  [unwired: 1 out]
              n189 = call "Client_email_addresses.vi"("Extra People to Email"=w496, "Contact All clients?"=w497) -> ()  [unwired: 1 in]
            }
            frame #3 {
              n190 = Unbundle By Name(w508) -> ("Ch Name"=w501:string)
              n191 = Build Array(w506) -> (w505:string[])
              n192 = Concatenate Strings(w500, w501) -> (w502:string)
              n193 = call "Email_Attachment_Plot.vi"("X axis name"="Time", "XY Graph"=w504, "Series Names"=w505, "message"=w507, "subject ([No Subject])"=w502) -> ()  [unwired: 1 in, 1 out]
            }
            frame #4 {
            }
          }
        }
        frame True {
        }
      }
      n194 = Concatenate Strings(w436, "") -> (w427:string)
      n195 = Select(t=0.0, s=w417, f=1.0) -> (s? t:f=w408:dbl)
      n196 = Select(t=w407, s=w409, f=w408) -> (s? t:f=w406:dbl)
    }
    frame "DRUCK" {
    }
    frame "GILL" {
      n197 = call "Gill_get_rdg.vi"("Channel Name"=w512, "Address"=w511) -> ("Output"=w514:dbl, "Status note"=w513:string)  [unwired: 2 in, 2 out]
    }
    frame "Hold Value" {
    }
    frame "IR2100" {
      n198 = call "IR2100_get_rdg.vi"("Address"=w517) -> ("Comment"=w519:string, "Reading"=w518:dbl)  [unwired: 2 in, 2 out]
    }
    frame "JEM" {
      n199 = Unbundle By Name(w536) -> ("Main"=w522:i32, "Ch."=w521:i32, "Port Name"=w531:string)
      n200 = case shown="0, Default" w521 {
        tunnel: [i16[] [-3, -2, -1, 0, 14, 29, 43, 57, 71, 86, 100] i16[] [0, 20, 40, 60, 80, 100, 120]] -> w525
        tunnel: [u8[] [10, 50, 80, 100, 120, 140, 160, 180, 200, 220, 240] u8[] [20, 50, 90, 130, 160, 200, 230]] -> w526
        frame 0, Default {
        }
        frame 1 {
        }
      }
      n201 = Add(x=w522, y=w521) -> (x+y=w520:i32)
      n202 = Threshold 1D Array(2:w532, 3:w525) -> (0:w528:dbl)  [unwired: 1 out]
      n203 = Round To Nearest(number=w528) -> (nearest integer value=w529:dbl)
      n204 = To Long Integer(number=w529) -> (32bit integer=w527:i32)
      n205 = Index Array(array=w526, index=w527) -> (element=w524:u8)
      n206 = call "DMX.vi"("Port Name"=w531, "DMX channel no."=w520, "Set value:"=w524, "Channel Name"=w535) -> ("error"=w530:bool)  [unwired: 2 out]
      n207 = Index Array(array=w525, index=w527) -> (element=w523:i16)
      n208 = case shown="False" w530 {
        tunnel: [w537 nan] -> w534
        tunnel: ["" "Comms Error"] -> w533
        tunnel: w523 -> [w539 _]
        frame False {
          n209 = To Double Precision Float(number=w539) -> (double precision float=w537:dbl)
        }
        frame True {
        }
      }
    }
    frame "LPA" {
      # "LPA was, IIRC, a serially-polled weighing platform we rented at Surrey for Athena Scaperdas' project at Atkins to weigh a helicopter with rotor running. \nTo add to the fun, it was RS232, so to make it addressable it was polled through an addressable ADAM 485-232 module"
      n210 = call "LPA400_get_rdg.vi"("Channel Name"=w548, "Address"=w549) -> ("Output"=w546:dbl, "Status note"=w547:string)  [unwired: 4 out]
    }
    frame "Oops", Default {
    }
    frame "PPT" {
      n211 = call "PPT_get_rdg.vi"("Channel Name"=w553, "Address"=w552) -> ("Reading"=w555:dbl, "Comment"=w554:string)  [unwired: 2 in, 2 out]
    }
    frame "Read A" {
      n212 = Unbundle By Name(w557) -> ("A"=w556:dbl)
    }
    frame "Read Ch" {
      n213 = Unbundle By Name(w562) -> ("String"=w559:string)
      n214 = call "Read_value_of_earlier_Ch.vi"("Desired Ch to Read"=w559, "Ch names"=w563, "Present scan array"=w564) -> ("Value"=w560:dbl, "Scan comment"=w561:string)  [unwired: 1 in]
    }
    frame "Run VI Named:" {
      n215 = Current VI's Path() -> (path=w583:path)
      n216 = Strip Path(path=w583) -> (stripped path=w584:path)  [unwired: 1 out]
      n217 = call <vilib>:"Trim Whitespace.vi"("string"=w566) -> ("trimmed string"=w565:string)  [unwired: 1 in]
      n218 = Strip Path(path=w584) -> (stripped path=w585:path)  [unwired: 1 out]
      n219 = Build Path(base path=w585, name or relative path="Run_vi_named") -> (appended path=w587:path)
      n220 = Build Path(base path=w587, name or relative path=w565) -> (appended path=w582:path)
      n221 = Open VI Reference(type specifier VI Refnum (for type only)=refnum<vi> refnum, vi path=w582) -> (vi reference=w578:refnum<vi>, error out=w577:errorcluster)  [unwired: 1 in, 3 out]
      n222 = property class="VI Interface Type 0"(reference=w578, error in=w577) -> (reference out=w580:refnum<vi>, error out=w579:errorcluster, "Front Panel Window:Open"=w581:bool)
      n223 = case shown="False" w581 {
        tunnel: w580 -> [w595 w597]
        tunnel: w579 -> [w594 w596]
        tunnel: [w593 w597] -> w576
        tunnel: [w591 w596] -> w575
        frame False {
          n224 = property class="VI Interface Type 0"(reference=w595, error in=w594, "Front Panel Window:Open"=TRUE) -> (reference out=w593:refnum<vi>, error out=w591:errorcluster)
        }
        frame True {
        }
      }
      n225 = call-by-ref "?"(reference=w576, error in=w575, "Scan Period"=w569, "Previous Scan Value"=w570, "Present scan array"=w571, "Value to Output"=w572, "Ch Description"=w573, "Ch names"=w574) -> (reference out=w589:refnum<vi>, error out=w590:errorcluster, "Scan comment"=w567:string, "Output"=w568:dbl)  [unwired: 2 in]
      n226 = Close Reference(reference=w589, error in (no error)=w590) -> ()  [unwired: 1 out]
    }
    frame "ScanPacer" {
      # "Uses a metronome to slow an otherwise over-fast scan table"
      n227 = call "ADAMPacer.vi"("Ch Description"=w600) -> ("Scan comment"=w598:string, "Output"=w599:dbl)  [unwired: 7 in]
    }
    frame "St Deviation" {
      # "The Channel names to average must appear in the comments field separated by semi colons"
      n228 = call "Get_array_values_fr_String.vi"("String Value"=w611) -> ("String array"=w610:string[])  [unwired: 1 out]
      n229 = Equal To 0?(x=w606) -> (x = 0?=w604:bool)
      n230 = case shown="False" w604 {
        tunnel: w605 -> [w617 _]
        tunnel: [w615 TRUE] -> w603
        tunnel: [w614 2.0 ("A")] -> w602
        frame False {
          n231 = Unbundle By Name(w617) -> ("D"=w614:dbl)
          n232 = Less?(x=w614, y=2.0) -> (x < y?=w615:bool)
        }
        frame True {
        }
      }
      n233 = global read "ADAM_Global.vi" "Active Ch names"() -> (w609:string[])
      n234 = case shown="False" w603 {
        tunnel: w613 -> [_ w652]
        tunnel: w612 -> [_ w651]
        tunnel: w610 -> [w622 w650]
        tunnel: [w620 w648] -> w601
        tunnel: w609 -> [_ w647]
        tunnel: [w623 w646] -> w608
        tunnel: w602 -> [w624 _]
        frame False {
          w631 = FALSE  # All Active Channels
          n235 = Get Date/Time In Seconds() -> (seconds since 1Jan1904=w634:timestamp)
          n236 = To Double Precision Float(number=w634) -> (double precision float=w632:dbl)
          n237 = Subtract(x=w632, y=w624) -> (x-y=w633:dbl)
          n238 = call "Get_ADAM_averages_server.vi"("No of averages"=1, "All Active Channels"=w631, "End time"=w632, "Start time"=w633, "Clients time"=w632, "ADAM Ch Names"=w622) -> ("DBL values"=w629:dbl[][])  [unwired: 4 out]
          n239 = Index Array(array=w629, index (row)=0) -> (element=w626:dbl[])  [unwired: 1 in]
          n240 = Array Subset(array=w626, index=1) -> (w625:dbl[])  [unwired: 1 in]
          n241 = for {
            tunnel: w625 -> [w640] mode=indexing
            tunnel: [w640] -> w623 mode=indexing if=w638
            tunnel: w622 -> [w637] mode=indexing
            shift-right: [w635] -> w620
            shift-left: "" -> [w636]
            n242 = Not A Number/Path/Refnum?(number/path/refnum=w640) -> (NaN/Path/Refnum?=w639:bool)
            n243 = Not(x=w639) -> (.not. x?=w638:bool)
            n244 = case shown="False" w638 {
              tunnel: w637 -> [w643 _]
              tunnel: w636 -> [w642 w645]
              tunnel: [w641 w645] -> w635
              frame False {
                n245 = Format Into String(format string="Channel \"%s\" is not currently active.\n", initial string=w642, w643) -> (resulting string=w641:string)  [unwired: 1 in, 1 out]
              }
              frame True {
              }
            }
          }
        }
        frame True {
          n246 = for {
            tunnel: w652 -> [w665]
            tunnel: w651 -> [w664]
            tunnel: w650 -> [w661] mode=indexing
            shift-right: [w662] -> w648
            shift-left: "" -> [w663]
            tunnel: [w655] -> w646 mode=indexing if=w653
            tunnel: w647 -> [w656]
            n247 = call "Read_value_of_earlier_Ch.vi"("Desired Ch to Read"=w661, "Ch names"=w665, "Present scan array"=w664) -> ("Value"=w659:dbl, "Scan comment"=w658:string)  [unwired: 1 in]
            n248 = Not A Number/Path/Refnum?(number/path/refnum=w659) -> (NaN/Path/Refnum?=w660:bool)
            n249 = case shown="False" w660 {
              tunnel: w661 -> [w668 _]
              tunnel: [w671 w681] -> w655
              tunnel: w659 -> [w670 w681]
              tunnel: [w673 w680] -> w657
              tunnel: w658 -> [w672 w680]
              tunnel: w656 -> [w669 _]
              frame False {
                n250 = Search 1D Array(1D array=w669, element=w668) -> (index of element=w666:i32)  [unwired: 1 in]
                n251 = Greater Or Equal To 0?(x=w666) -> (x >= 0?=w667:bool)
                n252 = case shown="False" w667 {
                  tunnel: w668 -> [w677 _]
                  tunnel: [w676 w679] -> w673
                  tunnel: w672 -> [_ w679]
                  tunnel: [nan w678] -> w671
                  tunnel: w670 -> [_ w678]
                  frame False {
                    n253 = Format Into String(format string="Channel \"%s\" is not currently active.\n", w677) -> (resulting string=w676:string)  [unwired: 2 in, 1 out]
                  }
                  frame True {
                  }
                }
              }
              frame True {
              }
            }
            n254 = Concatenate Strings(w663, w657) -> (w662:string)
            n255 = Not A Number/Path/Refnum?(number/path/refnum=w655) -> (NaN/Path/Refnum?=w654:bool)
            n256 = Not(x=w654) -> (.not. x?=w653:bool)
          }
        }
      }
      n257 = call <vilib>:"Std Deviation and Variance.vi"("X"=w608) -> ("standard deviation"=w607:dbl)  [unwired: 1 in, 2 out]
    }
    frame "Test" {
      w685 = 0.0005  # y
      n258 = Get Date/Time In Seconds() -> (seconds since 1Jan1904=w682:timestamp)
      n259 = To Double Precision Float(number=w682) -> (double precision float=w687:dbl)
      n260 = Subtract(x=w687, y=2969882881.0) -> (x-y=w686:dbl)
      n261 = Multiply(x=w686, y=w685) -> (x*y=w683:dbl)
      n262 = Random Number (0-1)() -> (number: 0 to 1=w684:dbl)
      n263 = Add(x=w684, y=w683) -> (x+y=w690:dbl)
    }
    frame "Thermistor" {
      n264 = call "4017_18_get_rdg.vi"("Channel Name"=w694, "Address"=w693) -> ("Reading"=w692:dbl, "Comment"=w695:string)  [unwired: 2 in, 2 out]
      n265 = call "Thermistor volts to temperature.vi"("V2 (V)"=w692) -> ("Temperature (degC)"=w691:dbl)
    }
    frame "Tracker" {
      n266 = while {
        tunnel: w701 -> [w725]
        tunnel: w700 -> [w724]
        tunnel: [w718] -> w699
        tunnel: w698 -> [w717]
        tunnel: [w711] -> w697
        tunnel: w696 -> [w710]
        i -> [w707]
        stop <- w704 continue-if-true
        n267 = Unbundle By Name(w724) -> ("Function"=w723:T3)
        n268 = Unbundle By Name(w725) -> ("Port Name"=w722:string, "Ch."=w713:i32, "Main"=w721:i32, "Sub"=w720:i32)
        n269 = case shown="\"Analogue Output\"" w723 {
          tunnel: [enum16{"Set", "Read"}."Set" ("Set") enum16{"Set", "Read"}."Set" ("Set") enum16{"Set", "Read"}."Set" ("Set") enum16{"Set", "Read"}."Set" ("Set") enum16{"Set", "Read"}."Set" ("Set") enum16{"Set", "Read"}."Read" ("Set") enum16{"Set", "Read"}."Read" ("Set")] -> w708
          tunnel: [enum16{"Logic", "Analogue"}."Analogue" ("Analogue") enum16{"Logic", "Analogue"}."Logic" ("Analogue") enum16{"Logic", "Analogue"}."Logic" ("Analogue") enum16{"Logic", "Analogue"}."Logic" ("Analogue") enum16{"Logic", "Analogue"}."Logic" ("Analogue") enum16{"Logic", "Analogue"}."Logic" ("Analogue") enum16{"Logic", "Analogue"}."Analogue" ("Analogue")] -> w719
          frame "Analogue Output" {
          }
          frame "Digital Output" {
          }
          frame "Relay Output" {
          }
          frame "Event rate" {
          }
          frame "Event counter" {
          }
          frame "Digital Input" {
          }
          frame "Analogue Input" {
          }
        }
        n270 = call "TalkTracker.vi"("PORT NAME"=w722, "Set"=w708, "Channel Name"=w717, "Value to set"=w710, "MODULE ADDRESS"=w721, "LOCATION"=w713, "NO. LOCATIONS"=w720, "Analogue"=w719) -> ("Response"=w715:string, "Good Set?"=w702:bool, "Comment out"=w718:string)  [unwired: 1 in, 4 out]
        n271 = Match Pattern(string=w715, regular expression="\r\n") -> (before substring=w714:string)  [unwired: 4 out]
        n272 = case shown="\"Set\"" w708 {
          tunnel: w714 -> [_ w737]
          tunnel: [w729 w736] -> w712
          tunnel: w710 -> [w731 _]
          tunnel: nan ("Reading") -> [w730 w735]
          tunnel: [w728 w733] -> w705
          tunnel: [0 ("y") 1 ("y")] -> w703
          tunnel: w702 -> [w726 _]
          frame "Set" {
            n273 = Not(x=w726) -> (.not. x?=w728:bool)
            n274 = Select(t=w731, s=w726, f=w730) -> (s? t:f=w729:dbl)
          }
          frame "Read" {
            n275 = String Length(string=w737) -> (length=w739:i32)
            n276 = Fract/Exp String To Number(string=w737, default (0 dbl)=w735) -> (offset past number=w740:i32, number=w738:dbl)  [unwired: 2 out]
            n277 = Equal?(x=w739, y=w740) -> (x = y?=w734:bool)
            n278 = Not(x=w734) -> (.not. x?=w733:bool)
            n279 = Select(t=w738, s=w734, f=w735) -> (s? t:f=w736:dbl)
          }
        }
        n280 = case shown="0, Default" w713 {
          tunnel: w712 -> [w741 w744]
          tunnel: [w741 w742] -> w711
          frame 0, Default {
          }
          frame 283 {
            n281 = Equal To 0?(x=w744) -> (x = 0?=w745:bool)
            n282 = Select(t=nan ("Reading"), s=w745, f=w744) -> (s? t:f=w742:dbl)
          }
        }
        n283 = Less?(x=w707, y=w703) -> (x < y?=w706:bool)
        n284 = And(x=w705, y=w706) -> (x .and. y?=w704:bool)
      }
    }
    frame "VICI" {
      n285 = To Long Integer(number=w772) -> (32bit integer=w767:i32)
      n286 = Unbundle By Name(w768) -> ("Port Name"=w770:string, "Ch."=w769:i32)
      n287 = call "Valco_Valve_Position.vi"("Channel Name"=w764, "Valve Number"=w769, "Port Name"=w770, "Requested Posn."=w767) -> ("Error Message"=w762:string, "Achieved Posn."=w765:T15)  [unwired: 2 out]
      n288 = Empty String/Path?(string/path=w762) -> ()  [unwired: 1 out]
      n289 = case shown="True" TRUE {
        tunnel: w768 -> [w779 _]
        tunnel: w767 -> [w778 _]
        tunnel: [w777 w809] -> w766
        tunnel: w765 -> [_ w809]
        tunnel: w764 -> [w776 _]
        tunnel: [w775 w808] -> w763
        tunnel: w762 -> [_ w808]
        tunnel: w762 -> [w774 _]
        tunnel: "X10" ("Port Name") -> [w773 _]
        frame False {
          n290 = stacked-sequence {
            tunnel: w779 -> [_ _ _ _ _ w800]
            tunnel: w778 -> [_ _ _ _ _ w796]
            tunnel: [_ _ _ _ _ w799] -> w777
            tunnel: w776 -> [_ _ _ _ _ w798]
            tunnel: [_ _ _ _ _ w797] -> w775
            tunnel: w774 -> [_ w785 _ _ _ _]
            tunnel: w773 -> [w780 _ _ w788 _ _]
            frame #0 {
              w782 = 3 items=["-----", "A", "B", "C", "D", "E", "F", "G", "H", "I", "J", "K", "L", "M", "N", "O", "P"] ("House Code")
              n291 = call "X10control.vi"("Port Name"=w780, "Power Request (ON)"=FALSE, "House Code"=w782, "Unit No."=5) -> ()  [unwired: 6 out]
            }
            frame #1 {
              n292 = call "Server_Emails.vi"("Message"=w785, "Contact All clients?"=TRUE, "Subject"="Powering Down FID Valve" ("Error Type")) -> ()  [unwired: 2 in, 3 out]
            }
            frame #2 {
              n293 = Wait (ms)(milliseconds to wait=u32 20000) -> ()  [unwired: 1 out]
            }
            frame #3 {
              w790 = 3 items=["-----", "A", "B", "C", "D", "E", "F", "G", "H", "I", "J", "K", "L", "M", "N", "O", "P"] ("House Code")
              n294 = call "X10control.vi"("Port Name"=w788, "Power Request (ON)"=TRUE, "House Code"=w790, "Unit No."=5) -> ()  [unwired: 6 out]
            }
            frame #4 {
              n295 = Wait (ms)(milliseconds to wait=u32 5000) -> ()  [unwired: 1 out]
            }
            frame #5 {
              n296 = Build Array(1 ("element"), 2 ("element"), w796) -> (w793:i32[])
              n297 = for {
                tunnel: w800 -> [w805]
                tunnel: [w804] -> w799
                tunnel: w798 -> [w803]
                tunnel: [w802] -> w797
                tunnel: w793 -> [w801] mode=indexing
                n298 = Unbundle By Name(w805) -> ("Port Name"=w806:string, "Ch."=w807:i32)
                n299 = call "Valco_Valve_Position.vi"("Channel Name"=w803, "Valve Number"=w807, "Port Name"=w806, "Requested Posn."=w801) -> ("Error Message"=w802:string, "Achieved Posn."=w804:T15)  [unwired: 2 out]
              }
            }
          }
        }
        frame True {
        }
      }
      n300 = To Double Precision Float(number=w766) -> (double precision float=w771:dbl)
    }
    frame "VIRTUAL" {
      n301 = case shown="\"EnFlo_Tunnel:Chilled Water:Valve Dem Pos\"" w815 {
        tunnel: [w829 w843 w857 w879 w894 w905 w919 w942 w970 w1054 w1064 w1085 w1190 w1216 w1243 w1263] -> w819
        tunnel: [w820 w849 w855 w883 w888 w903 w932 w951 w971 w1048 w1070 w1084 w1189 w1215 "" w1264] -> w818
        tunnel: w817 -> [w826 w851 w861 w885 w890 w908 w930 w953 w973 w1050 w1060 w1087 w1195 w1220 _ w1266]
        tunnel: w816 -> [w827 w850 w862 w884 w889 w909 w931 w952 w974 w1049 w1061 w1088 w1197 w1222 _ w1265]
        tunnel: w815 -> [w824 _ _ _ _ _ _ _ _ _ _ _ _ _ w1238 _]
        tunnel: w814 -> [w825 _ _ _ _ _ _ _ _ _ _ _ w1187 w1214 w1243 w1262]
        tunnel: w813 -> [w828 _ _ _ _ _ _ _ _ _ _ w1086 w1191 w1217 _ w1261]
        tunnel: w812 -> [_ _ w853 _ _ _ _ _ w975 _ _ w1089 _ _ _ _]
        tunnel: w811 -> [_ w842 _ _ _ w902 _ _ _ _ _ _ _ _ _ _]
        tunnel: w810 -> [_ _ _ _ _ _ _ _ _ _ _ _ _ _ _ _]
        frame "GMU:Remaining:", Default {
          n302 = Match Pattern(string=w824, regular expression="GMU:Remaining:" ("String to match")) -> (match substring=w822:string)  [unwired: 4 out]
          n303 = Empty String/Path?(string/path=w822) -> (empty?=w821:bool)
          n304 = case shown="False" w821 {
            tunnel: [w836 nan] -> w829
            tunnel: w828 -> [w835 _]
            tunnel: w827 -> [w834 _]
            tunnel: w826 -> [w833 _]
            tunnel: w825 -> [w832 _]
            tunnel: w824 -> [w831 _]
            tunnel: [w830 w838] -> w820
            frame False {
              n305 = call "Update_Rem_gas.vi"("Scan Period (s)"=w832, "Gas Remaining in"=w835, "Ch name"=w831, "Ch names"=w833, "Present scan array"=w834) -> ("Gas Remaining out"=w836:dbl, "Comments"=w830:string)  [unwired: 1 out]
            }
            frame True {
              n306 = Current VI's Path() -> (path=w840:path)
              n307 = Path To String(path=w840) -> (string=w839:string)
              n308 = Concatenate Strings(" was not matched in ", w839) -> (w838:string)
            }
          }
        }
        frame "GMU:Source:Meas Q" {
          n309 = call "Calculate_Release_Flowrates.vi"("Ch names"=w851, "Units"=enum16{"Q l/min", "M_dot Kg/min"}."Q l/min", "Present scan array"=w850) -> ("Trace"=w847:dbl, "Carrier"=w848:dbl, "Scan comments"=w849:string)
          n310 = Add(x=w848, y=w847) -> (x+y=w844:dbl)
          n311 = Not Equal To 0?(x=w844) -> (x != 0?=w845:bool)
          n312 = Select(t=w844, s=w845, f=w842) -> (s? t:f=w843:dbl)
        }
        frame "GMU:Detector:Strength" {
          n313 = Unbundle By Name(w853) -> ("C"=w852:dbl)
          n314 = call "Read_value_of_earlier_Ch.vi"("Desired Ch to Read"="GMU:Detector:Meas Current", "Ch names"=w861, "Present scan array"=w862) -> ("Value"=w858:dbl, "Scan comment"=w856:string)  [unwired: 1 in]
          n315 = Greater?(x=w858, y=w852) -> (0:w859:bool)
          n316 = case shown="True" w859 {
            tunnel: w853 -> [_ w874]
            tunnel: w858 -> [_ w869]
            tunnel: [100.0 ("Eng Values") w867] -> w857
            tunnel: ["Fault" w870] -> w854
            frame False {
            }
            frame True {
              n317 = Unbundle By Name(w874) -> ("D"=w865:dbl, "A"=w873:dbl, "B"=w872:dbl)
              n318 = Less?(x=w869, y=w865) -> (x < y?=w868:bool)
              n319 = Build Array(w873, w872) -> (w871:dbl[])
              n320 = call "Polynomial_convert.vi"("Calib constants"=w871, "Voltage"=w869) -> ("Eng Values"=w866:dbl)  [unwired: 4 out]
              n321 = case shown="True" w868 {
                tunnel: ["Saturated" ""] -> w870
                tunnel: [100.0 ("Eng Values") w877] -> w867
                tunnel: w866 -> [_ w877]
                frame False {
                }
                frame True {
                }
              }
            }
          }
          n322 = Concatenate Strings(w856, w854) -> (w855:string)
        }
        frame "GMU:Source:Meas M_dot" {
          n323 = call "Calculate_Release_Flowrates.vi"("Ch names"=w885, "Units"=enum16{"Q l/min", "M_dot Kg/min"}."M_dot Kg/min", "Present scan array"=w884) -> ("Trace"=w881:dbl, "Carrier"=w882:dbl, "Scan comments"=w883:string)
          n324 = Add(x=w882, y=w881) -> (x+y=w879:dbl)
        }
        frame "GMU:Source:Meas Density" {
          n325 = Build Array("GMU:Source:Meas M_dot", "GMU:Source:Meas Q") -> (w891:string[])
          n326 = call "Read_Earlier_Channels.vi"("Present scan array"=w889, "Ch names"=w890, "Desired Channels"=w891) -> ("Scan comments"=w888:string, "Index 0"=w887:dbl, "Index 1"=w886:dbl)  [unwired: 3 out]
          n327 = Not Equal To 0?(x=w887) -> (x != 0?=w895:bool)
          n328 = case shown="False" w895 {
            tunnel: w887 -> [_ w899]
            tunnel: w886 -> [_ w898]
            tunnel: [0.0 w897] -> w894
            frame False {
            }
            frame True {
              n329 = Divide(x=w899, y=w898) -> (x/y=w900:dbl)
              n330 = Multiply(x=w900, y=1000.0) -> (x*y=w897:dbl)
            }
          }
        }
        frame "GMU:Source:Meas Den Ratio" {
          n331 = call "Read_value_of_earlier_Ch.vi"("Desired Ch to Read"="GMU:Source:Meas Density", "Ch names"=w908, "Present scan array"=w909) -> ("Value"=w904:dbl, "Scan comment"=w903:string)  [unwired: 1 in]
          n332 = Equal?(x=w904, y=w902) -> (x = y?=w906:bool)
          n333 = case shown="False" w906 {
            tunnel: w904 -> [w911 _]
            tunnel: [w910 w916] -> w905
            tunnel: w902 -> [_ w916]
            frame False {
              n334 = global read "Gas_management_global.vi" "Release temp (deg C)"() -> (w914:dbl)
              n335 = global read "Gas_management_global.vi" "Atmos Pres (mbars)"() -> (w913:dbl)
              n336 = call "Gas_Density.vi"("Pressure (mbars)"=w913, "Temperature (deg C)"=w914, "Gas Name"="Air") -> ("Density Kg/m3"=w912:dbl)
              n337 = Divide(x=w911, y=w912) -> (x/y=w910:dbl)
            }
            frame True {
            }
          }
        }
        frame "GMU:Source:ppm/%Density" {
          # "Source ppm"
          # "% Delta Density of source"
          n338 = call "Read_value_of_earlier_Ch.vi"("Desired Ch to Read"="GMU:Source:Meas Strength", "Ch names"=w930, "Present scan array"=w931) -> ("Value"=w928:dbl, "Scan comment"=w932:string)  [unwired: 1 in]
          n339 = call "Read_value_of_earlier_Ch.vi"("Desired Ch to Read"="GMU:Source:Meas Den Ratio", "Ch names"=w930, "Present scan array"=w931) -> ("Value"=w926:dbl)  [unwired: 1 in, 1 out]
          n340 = Subtract(x=w926, y=1.0) -> (x-y=w923:dbl)
          n341 = Multiply(x=w928, y=10000.0) -> (x*y=w924:dbl)
          n342 = Multiply(x=w923, y=100.0) -> (x*y=w917:dbl)
          n343 = Absolute Value(x=w917) -> (abs(x)=w918:dbl)
          n344 = Greater?(x=w918, y=1.5) -> (0:w920:bool)
          n345 = case shown="False" w920 {
            tunnel: w924 -> [_ w937]
            tunnel: w917 -> [_ w936]
            tunnel: [nan w935] -> w919
            frame False {
            }
            frame True {
              n346 = Divide(x=w937, y=w936) -> (x/y=w935:dbl)
            }
          }
        }
        frame "GMU:Source:Meas Strength" {
          n347 = call "Calculate_Release_Flowrates.vi"("Ch names"=w953, "Units"=enum16{"Q l/min", "M_dot Kg/min"}."Q l/min", "Present scan array"=w952) -> ("Trace"=w945:dbl, "Carrier"=w946:dbl, "Scan comments"=w951:string)
          n348 = Equal To 0?(x=w946) -> (x = 0?=w948:bool)
          n349 = Equal To 0?(x=w945) -> (x = 0?=w949:bool)
          n350 = And(x=w948, y=w949) -> (x .and. y?=w947:bool)
          n351 = case shown="False" w947 {
            tunnel: w946 -> [w964 _]
            tunnel: w945 -> [w963 _]
            tunnel: [w962 0.0] -> w941
            frame False {
              n352 = Add(x=w964, y=w963) -> (x+y=w967:dbl)
              n353 = Divide(x=w963, y=w967) -> (x/y=w966:dbl)
              n354 = Multiply(x=w966, y=100.0) -> (x*y=w962:dbl)
            }
            frame True {
            }
          }
          n355 = while {
            tunnel: [w955] -> w938
            tunnel: [w956] -> w940
            tunnel: w941 -> [w961]
            shift-left: _ -> [w955]
            shift-left: _ -> [w960]
            shift-right: [w961] -> _
            stop <- FALSE continue-if-true
            w959 = 6.0 ("y")
            n356 = Less?(x=w960, y=w959) -> (x < y?=w958:bool)
            n357 = Less?(x=w955, y=w959) -> (x < y?=w957:bool)
            n358 = Or(x=w958, y=w957) -> (x .or. y?=w956:bool)
          }
          n359 = Greater?(x=w941, y=7.0) -> (0:w939:bool)
          n360 = And(x=w940, y=w939) -> (x .and. y?=w943:bool)
          n361 = Select(t=w938, s=w943, f=w941) -> (s? t:f=w942:dbl)
        }
        frame "EnFlo_Tunnel:Inlet_Temp:St Deviation" {
          n362 = global read "ADAM_Global.vi" "Active Ch names"() -> (w979:string[])
          n363 = Unbundle By Name(w975) -> ("A"=w976:dbl)
          n364 = Less?(x=w976, y=2.0) -> (x < y?=w977:bool)
          n365 = case shown="True" w977 {
            tunnel: w973 -> [_ w1015]
            tunnel: w974 -> [_ w1014]
            tunnel: string[] ["EnFlo_Tunnel:Inlet_Y=-1500:Z=50", "EnFlo_Tunnel:Inlet_Y=-1000:Z=50", "EnFlo_Tunnel:Inlet_Y=-500:Z=50", "EnFlo_Tunnel:Temp:Inlet_15_Bottom", "EnFlo_Tunnel:Inlet_Y=500:Z=50", "EnFlo_Tunnel:Inlet_Y=1000:Z=50", "EnFlo_Tunnel:Inlet_Y=1500:Z=50", "EnFlo_Tunnel:Inlet_Y=-1500:Z=450", "EnFlo_Tunnel:Inlet_Y=-1000:Z=450", "EnFlo_Tunnel:Inlet_Y=-500:Z=450", "EnFlo_Tunnel:Temp:Inlet_11", "EnFlo_Tunnel:Inlet_Y=500:Z=450", "EnFlo_Tunnel:Inlet_Y=1000:Z=450", "EnFlo_Tunnel:Inlet_Y=1500:Z=450", "EnFlo_Tunnel:Inlet_Y=-1500:Z=950", "EnFlo_Tunnel:Inlet_Y=-1000:Z=950", "EnFlo_Tunnel:Inlet_Y=-500:Z=950", "EnFlo_Tunnel:Temp:Inlet_6", "EnFlo_Tunnel:Inlet_Y=500:Z=950", "EnFlo_Tunnel:Inlet_Y=1000:Z=950", "EnFlo_Tunnel:Inlet_Y=1500:Z=950", "EnFlo_Tunnel:Inlet_Y=-1500:Z=1450", "EnFlo_Tunnel:Inlet_Y=-1000:Z=1450", "EnFlo_Tunnel:Inlet_Y=-500:Z=1450", "EnFlo_Tunnel:Temp:Inlet_1_Top", "EnFlo_Tunnel:Inlet_Y=500:Z=1450", "EnFlo_Tunnel:Inlet_Y=1000:Z=1450", "EnFlo_Tunnel:Inlet_Y=1500:Z=1450", "EnFlo_Tunnel:Setpoint:Inlet_15_Bottom", "EnFlo_Tunnel:Setpoint:Inlet_11", "EnFlo_Tunnel:Setpoint:Inlet_6", "EnFlo_Tunnel:Setpoint:Inlet_1_Top"] ("subarray") -> [w984 w1013]
            tunnel: [w982 w1011] -> w971
            tunnel: w979 -> [_ w1010]
            tunnel: [w985 w1007] -> w969
            tunnel: w976 -> [w986 _]
            frame False {
              w992 = FALSE  # All Active Channels
              n366 = Get Date/Time In Seconds() -> (seconds since 1Jan1904=w995:timestamp)
              n367 = To Double Precision Float(number=w995) -> (double precision float=w993:dbl)
              n368 = Subtract(x=w993, y=w986) -> (x-y=w994:dbl)
              n369 = call "Get_ADAM_averages_server.vi"("No of averages"=1, "All Active Channels"=w992, "End time"=w993, "Start time"=w994, "Clients time"=w993, "ADAM Ch Names"=w984) -> ("DBL values"=w990:dbl[][])  [unwired: 4 out]
              n370 = Index Array(array=w990, index (row)=0) -> (element=w987:dbl[])  [unwired: 1 in]
              n371 = Array Subset(array=w987, index=1) -> (w981:dbl[])  [unwired: 1 in]
              n372 = call "Normalise Inlet Temps array.vi"("Temps plus setpoints"=w981) -> ("Normalised Temps"=w980:dbl[])
              n373 = for {
                tunnel: w980 -> [w1001] mode=indexing
                tunnel: [w1001] -> w985 mode=indexing if=w999
                tunnel: w984 -> [w998] mode=indexing
                shift-right: [w996] -> w982
                shift-left: "" -> [w997]
                n374 = Not A Number/Path/Refnum?(number/path/refnum=w1001) -> (NaN/Path/Refnum?=w1000:bool)
                n375 = Not(x=w1000) -> (.not. x?=w999:bool)
                n376 = case shown="False" w999 {
                  tunnel: w998 -> [w1004 _]
                  tunnel: w997 -> [w1003 w1006]
                  tunnel: [w1002 w1006] -> w996
                  frame False {
                    n377 = Format Into String(format string="Channel \"%s\" is not currently active.\n", initial string=w1003, w1004) -> (resulting string=w1002:string)  [unwired: 1 in, 1 out]
                  }
                  frame True {
                  }
                }
              }
            }
            frame True {
              n378 = for {
                tunnel: w1015 -> [w1029]
                tunnel: w1014 -> [w1028]
                tunnel: w1013 -> [w1025] mode=indexing
                shift-right: [w1026] -> w1011
                shift-left: "" -> [w1027]
                tunnel: w1010 -> [w1020]
                tunnel: [w1019] -> w1009 mode=indexing
                n379 = call "Read_value_of_earlier_Ch.vi"("Desired Ch to Read"=w1025, "Ch names"=w1029, "Present scan array"=w1028) -> ("Value"=w1023:dbl, "Scan comment"=w1022:string)  [unwired: 1 in]
                n380 = Not A Number/Path/Refnum?(number/path/refnum=w1023) -> (NaN/Path/Refnum?=w1024:bool)
                n381 = case shown="False" w1024 {
                  tunnel: w1025 -> [w1032 _]
                  tunnel: [w1035 w1045] -> w1019
                  tunnel: w1023 -> [w1034 w1045]
                  tunnel: [w1037 w1044] -> w1021
                  tunnel: w1022 -> [w1036 w1044]
                  tunnel: w1020 -> [w1033 _]
                  frame False {
                    n382 = Search 1D Array(1D array=w1033, element=w1032) -> (index of element=w1030:i32)  [unwired: 1 in]
                    n383 = Greater Or Equal To 0?(x=w1030) -> (x >= 0?=w1031:bool)
                    n384 = case shown="False" w1031 {
                      tunnel: w1032 -> [w1041 _]
                      tunnel: [w1040 w1043] -> w1037
                      tunnel: w1036 -> [_ w1043]
                      tunnel: [nan w1042] -> w1035
                      tunnel: w1034 -> [_ w1042]
                      frame False {
                        n385 = Format Into String(format string="Channel \"%s\" is not currently active.\n", w1041) -> (resulting string=w1040:string)  [unwired: 2 in, 1 out]
                      }
                      frame True {
                      }
                    }
                  }
                  frame True {
                  }
                }
                n386 = Concatenate Strings(w1027, w1021) -> (w1026:string)
              }
              n387 = call "Normalise Inlet Temps array.vi"("Temps plus setpoints"=w1009) -> ("Normalised Temps"=w1008:dbl[])
              n388 = for {
                tunnel: w1008 -> [w1017] mode=indexing
                tunnel: [w1017] -> w1007 mode=indexing if=w1016
                n389 = Not A Number/Path/Refnum?(number/path/refnum=w1017) -> (NaN/Path/Refnum?=w1018:bool)
                n390 = Not(x=w1018) -> (.not. x?=w1016:bool)
              }
            }
          }
          n391 = call <vilib>:"Std Deviation and Variance.vi"("X"=w969) -> ("standard deviation"=w970:dbl)  [unwired: 1 in, 2 out]
        }
        frame "EnFlo Lab:labstrat1:Delta T" {
          n392 = Build Array("EnFlo Lab:labstrat1:Z=4.5m", "EnFlo Lab:labstrat1:Z=0.5m") -> (w1053:string[])
          n393 = call "Read_Earlier_Channels.vi"("Present scan array"=w1049, "Ch names"=w1050, "Desired Channels"=w1053) -> ("Scan comments"=w1048:string, "Index 0"=w1047:dbl, "Index 1"=w1046:dbl)  [unwired: 3 out]
          n394 = Subtract(x=w1047, y=w1046) -> (x-y=w1054:dbl)
        }
        frame "EnFlo_Tunnel:Inlet:K_Factor" {
          n395 = call "Read_value_of_earlier_Ch.vi"("Desired Ch to Read"="EnFlo_Tunnel:Speed:Dem Velocity", "Ch names"=w1060, "Present scan array"=w1061) -> ("Value"=w1056:dbl)  [unwired: 1 in, 1 out]
          n396 = Build Array("EnFlo_Tunnel:Pressure:Static", "EnFlo_Tunnel:Reference:Velocity", "Froude:NPL:Atmos_Press", "EnFlo_Tunnel:Inlet_Temp:Average") -> (w1073:string[])
          n397 = call "Read_Earlier_Channels.vi"("Present scan array"=w1061, "Ch names"=w1060, "Desired Channels"=w1073) -> ("Scan comments"=w1070:string, "Index 0"=w1065:dbl, "Index 1"=w1063:dbl, "Index 2"=w1066:dbl, "Index 3"=w1067:dbl)  [unwired: 1 out]
          n398 = Greater?(x=w1063, y=0.8) -> (0:w1058:bool)
          n399 = while {
            shift-right: [w1077] -> _
            shift-left: _ -> [_]
            shift-left: _ -> [_]
            shift-left: _ -> [_]
            shift-left: _ -> [_]
            shift-left: _ -> [_]
            shift-left: _ -> [_]
            shift-left: _ -> [_]
            shift-left: _ -> [_]
            shift-left: _ -> [_]
            shift-left: _ -> [_]
            shift-left: _ -> [w1076]
            tunnel: w1056 -> [w1077]
            tunnel: [w1075] -> w1055
            stop <- TRUE stop-if-true
            n400 = Equal?(x=w1077, y=w1076) -> (x = y?=w1075:bool)
          }
          n401 = And(x=w1055, y=w1058) -> (x .and. y?=w1057:bool)
          n402 = case shown="True" w1057 {
            tunnel: w1067 -> [_ w1083]
            tunnel: w1066 -> [_ w1082]
            tunnel: w1063 -> [_ w1081]
            tunnel: w1065 -> [_ w1080]
            tunnel: [nan w1079] -> w1064
            frame False {
            }
            frame True {
              n403 = formula code="Rho=(Patmos*100)/(287*(T+273));\nDyn_Pres=0.5*Rho*U*U;\nK=(-Pstatic/Dyn_Pres)-1;"("Pstatic"=w1080, "Patmos"=w1082, "T"=w1083, "U"=w1081) -> ("K"=w1079:dbl)  [unwired: 2 out]
            }
          }
        }
        frame "EnFlo_Tunnel:Chilled Water:Valve Dem Pos" {
          n404 = while {
            shift-right: [w1097] -> _
            shift-left: _ -> [w1099]
            tunnel: w1089 -> [w1098]
            tunnel: w1088 -> [w1096]
            tunnel: w1087 -> [w1095]
            tunnel: w1086 -> [w1094]
            tunnel: [w1093] -> w1085
            tunnel: [w1092] -> w1084
            shift-right: [w1091] -> _
            shift-left: _ -> [w1090]
            stop <- TRUE stop-if-true
            # "Current"
            # "Dem"
            # "Run PID"
            n405 = stacked-sequence {
              seq-local: [w1110 _ _] -> [_ _ w1134]
              seq-local: [_ w1119 _] -> [_ _ w1131]
              seq-local: [_ w1118 _] -> [_ _ w1128]
              seq-local: [_ w1117 _] -> [_ _ w1127]
              seq-local: [w1101 _ _] -> [_ _ w1125]
              tunnel: w1099 -> [w1108 _ _]
              tunnel: w1098 -> [w1115 _ _]
              tunnel: [w1107 _ _] -> w1097
              tunnel: w1096 -> [_ w1124 w1133]
              tunnel: w1095 -> [_ w1123 w1132]
              tunnel: w1094 -> [w1103 _ w1130]
              tunnel: [_ _ w1129] -> w1093
              tunnel: [_ _ w1126] -> w1092
              tunnel: [w1105 _ _] -> w1091
              tunnel: w1090 -> [w1104 _ _]
              frame #0 {
                n406 = Get Date/Time In Seconds() -> (seconds since 1Jan1904=w1116:timestamp)
                n407 = Unbundle By Name(w1115) -> ("A"=w1114:dbl)
                n408 = To Double Precision Float(number=w1116) -> (double precision float=w1109:dbl)
                n409 = Build Array (concatenate)(w1104, w1103) -> (w1102:dbl[])
                n410 = Subtract(x=w1109, y=w1108) -> (x-y=w1113:dbl)
                n411 = Greater?(x=w1113, y=w1114) -> (0:w1112:bool)
                n412 = Not A Number/Path/Refnum?(number/path/refnum=w1113) -> (NaN/Path/Refnum?=w1111:bool)
                n413 = call-poly <vilib>:"Mean.vi"("X"=w1102) -> ("mean"=w1101:dbl)  [unwired: 1 out]
                n414 = Or(x=w1111, y=w1112) -> (x .or. y?=w1110:bool)
                n415 = Select(t=w1109, s=w1110, f=w1108) -> (s? t:f=w1107:dbl)
                n416 = Array Subset(array=w1102, length="History Length") -> (w1105:dbl[])  [unwired: 1 in]
              }
              frame #1 {
                n417 = Build Array("EnFlo_Tunnel:Chilled Water:Dem Temp", "EnFlo_Tunnel:Chilled Water:Supply") -> (w1120:string[])
                n418 = call "Read_Earlier_Channels.vi"("Present scan array"=w1124, "Ch names"=w1123, "Desired Channels"=w1120) -> ("Scan comments"=w1117:string, "Index 0"=w1119:dbl, "Index 1"=w1118:dbl)  [unwired: 3 out]
              }
              frame #2 {
                n419 = case shown="True" w1134 {
                  tunnel: w1133 -> [_ w1154]
                  tunnel: w1132 -> [_ w1153]
                  tunnel: w1131 -> [_ w1151]
                  tunnel: w1130 -> [w1136 w1150]
                  tunnel: [w1136 w1146] -> w1129
                  tunnel: w1128 -> [_ w1145]
                  tunnel: w1127 -> [w1135 w1144]
                  tunnel: [w1135 w1142] -> w1126
                  tunnel: w1125 -> [_ w1137]
                  frame False {
                  }
                  frame True {
                    n420 = call "Read_Earlier_Channels.vi"("Present scan array"=w1154, "Ch names"=w1153, "Desired Channels"=string[] ["EnFlo_Tunnel:Chiller_Pump:Running", "EnFlo_Tunnel:Chiller_Pump:Enable", "Uni:Chilled Water:Temp"] ("appended array")) -> ("Scan comments"=w1143:string, "Index 0"=w1139:dbl, "Index 1"=w1147:dbl, "Index 2"=w1138:dbl)  [unwired: 2 out]
                    n421 = Greater?(x=w1147, y=0.5) -> (0:w1148:bool)
                    n422 = Greater?(x=w1139, y=0.5) -> (0:w1140:bool)
                    n423 = case shown="True" w1140 {
                      tunnel: [w1167 w1183] -> w1146
                      tunnel: w1151 -> [_ w1176]
                      tunnel: w1145 -> [_ w1184]
                      tunnel: w1148 -> [w1158 _]
                      tunnel: w1150 -> [_ w1175]
                      tunnel: w1138 -> [_ w1177]
                      tunnel: w1137 -> [_ w1171]
                      frame False {
                        n424 = Seconds To Date/Time() -> (date time rec=w1155:T16)  [unwired: 2 out]
                        n425 = Unbundle By Name(w1155) -> ("day of week"=w1162:i32, "hour"=w1164:i32)
                        n426 = Less?(x=w1164, y=3) -> (x < y?=w1159:bool)
                        n427 = Equal?(x=7, y=w1162) -> (x = y?=w1160:bool)
                        n428 = And(x=w1160, y=w1159) -> (x .and. y?=w1157:bool)
                        n429 = case shown="True" w1158 {
                          tunnel: w1157 -> [w1168 w1170]
                          tunnel: [w1168 w1169] -> w1156
                          frame False {
                          }
                          frame True {
                            n430 = Not(x=w1170) -> (.not. x?=w1169:bool)
                          }
                        }
                        n431 = Select(t=0.0, s=w1156, f=100.0) -> (s? t:f=w1167:dbl)
                      }
                      frame True {
                        w1185 = 100.0  # Max
                        w1186 = 0.0  # Min
                        n432 = call "PID.vi"("Present Value"=w1184, "Previous Scan Value"=w1175, "Setpoint"=w1176) -> ("Dem Output"=w1182:dbl)
                        n433 = Divide(x=w1171, y=100.0) -> (x/y=w1172:dbl)
                        n434 = Subtract(x=w1177, y=8.5) -> (x-y=w1178:dbl)
                        n435 = Compound Arithmetic op=MULTIPLY(w1178, w1172, "K_Uni_chilled water") -> (w1179:dbl)
                        n436 = Add(x=w1182, y=w1179) -> (x+y=w1181:dbl)
                        n437 = In Range and Coerce(upper limit=w1185, x=w1181, lower limit=w1186) -> (coerced(x)=w1183:dbl)  [unwired: 1 out]
                      }
                    }
                    n438 = Concatenate Strings(w1143, w1144) -> (w1142:string)
                  }
                }
              }
            }
          }
        }
        frame "EnFlo_Tunnel:Hydrosonic:Integral" {
          n439 = Build Array("EnFlo_Tunnel:Reference:Velocity", "Hydrosonic:Transducer:Setting") -> (w1196:string[])
          n440 = call "Read_Earlier_Channels.vi"("Present scan array"=w1197, "Ch names"=w1195, "Desired Channels"=w1196) -> ("Scan comments"=w1189:string, "Index 0"=w1194:dbl, "Index 1"=w1188:dbl)  [unwired: 3 out]
          n441 = Greater?(x=w1194, y=0.5) -> (0:w1192:bool)
          n442 = case shown="True" w1192 {
            tunnel: w1191 -> [w1200 w1208]
            tunnel: [w1200 w1207] -> w1190
            tunnel: w1188 -> [_ w1206]
            tunnel: w1187 -> [_ w1205]
            frame False {
            }
            frame True {
              w1203 = 8640000.0  # Seconds per day x 100
              n443 = Multiply(x=w1206, y=w1205) -> (x*y=w1204:dbl)
              n444 = Divide(x=w1204, y=w1203) -> (x/y=w1202:dbl)
              n445 = Not A Number/Path/Refnum?(number/path/refnum=w1202) -> (NaN/Path/Refnum?=w1201:bool)
              n446 = case shown="False" w1201 {
                tunnel: w1208 -> [w1211 w1212]
                tunnel: [w1210 w1212] -> w1207
                tunnel: w1202 -> [w1209 _]
                frame False {
                  n447 = Add(x=w1209, y=w1211) -> (x+y=w1210:dbl)
                }
                frame True {
                }
              }
            }
          }
        }
        frame "EnFlo_Tunnel:Days Run at:2.5m/s" {
          n448 = Build Array("EnFlo_Tunnel:Reference:Velocity") -> (w1221:string[])
          n449 = call "Read_Earlier_Channels.vi"("Present scan array"=w1222, "Ch names"=w1220, "Desired Channels"=w1221) -> ("Scan comments"=w1215:string, "Index 0"=w1213:dbl)  [unwired: 4 out]
          n450 = Greater?(x=w1213, y=0.5) -> (0:w1218:bool)
          n451 = case shown="True" w1218 {
            tunnel: w1217 -> [w1224 w1232]
            tunnel: [w1224 w1231] -> w1216
            tunnel: w1213 -> [_ w1230]
            tunnel: w1214 -> [_ w1229]
            frame False {
            }
            frame True {
              w1227 = 216000.0  # Seconds per day x 2.5
              n452 = Multiply(x=w1230, y=w1229) -> (x*y=w1228:dbl)
              n453 = Divide(x=w1228, y=w1227) -> (x/y=w1226:dbl)
              n454 = Not A Number/Path/Refnum?(number/path/refnum=w1226) -> (NaN/Path/Refnum?=w1225:bool)
              n455 = case shown="True" w1225 {
                tunnel: w1232 -> [w1235 w1236]
                tunnel: [w1234 w1236] -> w1231
                tunnel: w1226 -> [w1233 _]
                frame False {
                  n456 = Add(x=w1233, y=w1235) -> (x+y=w1234:dbl)
                }
                frame True {
                }
              }
            }
          }
        }
        frame "Complete:Scan:Period" {
          n457 = while {
            tunnel: [w1246] -> w1239
            tunnel: [w1253] -> w1241
            shift-left: _ -> [w1253]
            shift-right: [w1254] -> w1242
            tunnel: w1238 -> [w1250]
            tunnel: [w1245] -> w1237
            stop <- FALSE continue-if-true
            w1245 = 10.0 ("Averaging time (mins)")
            n458 = Build Array(w1250) -> (w1249:string[])
            n459 = call "Get_Channel_averages.vi"("Desired Ch Names"=w1249, "Averaging time (mins)"=w1245) -> ("number"=w1248:dbl[])  [unwired: 1 in, 2 out]
            n460 = Index Array(array=w1248, index=0) -> (element=w1246:dbl)
            n461 = Greater?(x=w1246, y=20.0) -> (0:w1254:bool)
          }
          n462 = Compound Arithmetic op=AND(w1242, invert w1241) -> (w1240:bool)
          n463 = case shown="True" w1240 {
            tunnel: w1239 -> [_ w1260]
            tunnel: w1237 -> [_ w1255]
            frame False {
            }
            frame True {
              n464 = Format Into String(format string="Warning! The average scan period on the ADAM Scan table is %.1f seconds over the last %d minutes." ("Format String"), w1260, w1255) -> (resulting string=w1258:string)  [unwired: 2 in, 1 out]
              n465 = call "Server_Emails.vi"("Message"=w1258, "Contact All clients?"=TRUE, "Subject"="Scan Period") -> ()  [unwired: 2 in, 3 out]
            }
          }
        }
        frame "GMU:Source:Est Time" {
          # "NaN's"
          # "Est?"
          # "Inband?"
          n466 = stacked-sequence {
            seq-local: [w1267 _ _ _] -> [_ _ w1314 _]
            seq-local: [_ w1279 _ _] -> [_ _ w1311 _]
            seq-local: [_ w1280 _ _] -> [_ _ w1309 _]
            seq-local: [_ _ w1316 _] -> [_ _ _ w1332]
            seq-local: [w1271 _ _ _] -> [_ _ w1313 _]
            seq-local: [_ w1278 _ _] -> [_ _ _ w1328]
            tunnel: w1266 -> [w1273 w1281 w1319 _]
            tunnel: w1265 -> [w1272 w1282 w1320 _]
            tunnel: [_ _ w1312 _] -> w1264
            tunnel: [_ _ _ w1331] -> w1263
            tunnel: w1262 -> [_ _ _ w1330]
            tunnel: w1261 -> [_ _ _ w1329]
            frame #0 {
              n467 = Build Array("GMU:Carrier 1:Dem Q", "GMU:Carrier 2:Dem Q", "GMU:Trace:Dem Q") -> (w1274:string[])
              n468 = call "Read_Earlier_Channels.vi"("Present scan array"=w1272, "Ch names"=w1273, "Desired Channels"=w1274) -> ("Scan comments"=w1271:string, "Index 0"=w1270:dbl, "Index 1"=w1269:dbl, "Index 2"=w1268:dbl)  [unwired: 2 out]
              n469 = Build Array(w1270, w1269, w1268) -> (w1267:dbl[])
            }
            frame #1 {
              n470 = for {
                N: 2 -> [_]
                tunnel: w1282 -> [w1292]
                tunnel: w1281 -> [w1293]
                tunnel: [w1291] -> w1279 mode=indexing
                tunnel: [w1298] -> w1280 mode=indexing
                tunnel: [w1297] -> w1278 mode=indexing
                i -> [w1303]
                w1302 = 23.0  # %
                n471 = case shown="0, Default" w1303 {
                  tunnel: ["GMU:Source:Meas Q" "GMU:Source:Meas Strength"] -> w1296
                  tunnel: ["GMU:Source:Dem Q" "GMU:Source:Dem Strength"] -> w1295
                  frame 0, Default {
                  }
                  frame 1 {
                  }
                }
                n472 = Build Array(w1295, w1296) -> (w1294:string[])
                n473 = call "Read_Earlier_Channels.vi"("Present scan array"=w1292, "Ch names"=w1293, "Desired Channels"=w1294) -> ("Scan comments"=w1291:string, "Index 0"=w1289:dbl, "Index 1"=w1290:dbl)  [unwired: 3 out]
                n474 = Not A Number/Path/Refnum?(number/path/refnum=w1290) -> (NaN/Path/Refnum?=w1297:bool)
                n475 = Subtract(x=w1290, y=w1289) -> (x-y=w1288:dbl)
                n476 = Greater Than 0?(x=w1289) -> (x > 0?=w1299:bool)
                n477 = Less?(x=w1288, y=0.05) -> (x < y?=w1285:bool)
                n478 = call "In_Range_check.vi"("%"=w1302, "Mode"=In_Range."%", "Value"=w1290, "Setpoint"=w1289) -> ("In Range"=w1286:bool)  [unwired: 1 in, 2 out]
                n479 = Or(x=w1286, y=w1285) -> (x .or. y?=w1284:bool)
                n480 = And(x=w1284, y=w1299) -> (x .and. y?=w1300:bool)
                n481 = Compound Arithmetic op=OR(w1300, invert w1299, w1297) -> (w1298:bool)
              }
            }
            frame #2 {
              n482 = while {
                tunnel: [w1327] -> w1315
                tunnel: w1314 -> [w1326]
                shift-left: _ -> [w1327]
                shift-right: [w1326] -> _
                stop <- FALSE continue-if-true
              }
              n483 = Equal?(x=w1314, y=w1315) -> (x = y?=w1321:bool)
              n484 = call "Read_value_of_earlier_Ch.vi"("Desired Ch to Read"="GMU:Source:Dem Q", "Ch names"=w1319, "Present scan array"=w1320) -> ("Value"=w1317:dbl)  [unwired: 1 in, 1 out]
              n485 = Greater Than 0?(x=w1317) -> (x > 0?=w1324:bool)
              n486 = And Array Elements(Boolean array=w1309) -> (logical AND=w1308:bool)
              n487 = Select(t=w1308, s=w1324, f=TRUE) -> (s? t:f=w1322:bool)
              n488 = Compound Arithmetic op=AND(w1321, w1322) -> (w1316:bool)
              n489 = Concatenate Strings(w1311) -> (w1310:string)
              n490 = Concatenate Strings(w1310, w1313) -> (w1312:string)
            }
            frame #3 {
              n491 = case shown="False" w1332 {
                tunnel: [0.0 w1334] -> w1331
                tunnel: w1330 -> [_ w1339]
                tunnel: w1329 -> [_ w1335]
                tunnel: w1328 -> [_ w1338]
                frame False {
                }
                frame True {
                  n492 = Or Array Elements(Boolean array=w1338) -> (logical OR=w1337:bool)
                  n493 = Add(x=w1339, y=w1335) -> (x+y=w1336:dbl)
                  n494 = Select(t=w1335, s=w1337, f=w1336) -> (s? t:f=w1334:dbl)
                }
              }
            }
          }
        }
      }
    }
    frame "Vaisala" {
      n495 = Unbundle By Name(w1346) -> ("Main"=w1342:i32, "Ch."=w1343:i32, "Port Name"=w1344:string)
      n496 = call "HMP231.vi"("Channel Name"=w1345, "Port Name"=w1344, "Channel"=w1343, "Address"=w1342) -> ("Output"=w1340:dbl, "Status note"=w1341:string)  [unwired: 2 out]
    }
    frame "WEST" {
    }
    frame "Web Client" {
      w1358 = 7200.0  # 2 Hours in Seconds
      n497 = Concatenate Strings(w1367, ":Last read" ("Substring")) -> (w1365:string)
      n498 = call "Remember_value.vi"("Mode"=Remember_value_mode."Read only", "Ch name"=w1365) -> ("Output Value"=w1364:dbl)  [unwired: 1 in]
      n499 = Not A Number/Path/Refnum?(number/path/refnum=w1364) -> (NaN/Path/Refnum?=w1362:bool)
      n500 = Get Date/Time In Seconds() -> (seconds since 1Jan1904=w1357:timestamp)
      n501 = To Double Precision Float(number=w1357) -> (double precision float=w1355:dbl)
      n502 = Subtract(x=w1355, y=w1364) -> (x-y=w1370:dbl)
      n503 = Greater?(x=w1370, y=1800.0) -> (0:w1363:bool)
      n504 = Or(x=w1363, y=w1362) -> (x .or. y?=w1349:bool)
      n505 = case shown="True" w1349 {
        frame False {
        }
        frame True {
          n506 = global read "Constants_global.vi" "EnFlo SW Folder"() -> (w1373:path)
          n507 = Build Path(base path=w1373, name or relative path=path "ADAM Server/Sub VI's/Web_Client.vi") -> (appended path=w1372:path)
          n508 = Open VI Reference(vi path=w1372) -> (vi reference=w1377:refnum<vi>, error out=w1378:errorcluster)  [unwired: 1 in, 4 out]
          n509 = property class="VI"(reference=w1377, error in=w1378) -> (reference out=w1380:refnum<vi>, error out=w1381:errorcluster, "Front Panel Window:Open"=w1379:bool)
          n510 = case shown="False" w1379 {
            tunnel: w1380 -> [w1387 w1390]
            tunnel: w1381 -> [w1386 w1389]
            tunnel: [w1385 w1390] -> w1382
            tunnel: [w1384 w1389] -> w1383
            frame False {
              n511 = property class="VI"(reference=w1387, error in=w1386, "Front Panel Window:Open"=TRUE) -> (reference out=w1385:refnum<vi>, error out=w1384:errorcluster)
            }
            frame True {
            }
          }
          n512 = invoke class="VI" method="Run VI"(reference=w1382, error in=w1383, "Wait until done"=FALSE, "Auto Dispose Ref"=TRUE) -> ()  [unwired: 1 in, 5 out]
        }
      }
      n513 = Concatenate Strings(w1367, ":value time" ("Substring")) -> (w1351:string)
      n514 = call "Remember_value.vi"("Mode"=Remember_value_mode."Read only", "Ch name"=w1367) -> ("Output Value"=w1371:dbl)  [unwired: 1 in]
      n515 = call "Remember_value.vi"("Mode"=Remember_value_mode."Read only", "Ch name"=w1351) -> ("Output Value"=w1356:dbl)  [unwired: 1 in]
      n516 = Subtract(x=w1355, y=w1356) -> (x-y=w1354:dbl)
      n517 = Greater?(x=w1354, y=w1358) -> (0:w1361:bool)
      n518 = case shown="True" w1361 {
        tunnel: w1354 -> [_ w1396]
        tunnel: 3600.0 ("y") -> [_ w1395]
        tunnel: ["" w1393] -> w1360
        frame False {
        }
        frame True {
          n519 = Divide(x=w1396, y=w1395) -> (x/y=w1392:dbl)
          n520 = Format Into String(format string="Value is %d hours old." ("Format String"), w1392) -> (resulting string=w1393:string)  [unwired: 2 in, 1 out]
        }
      }
    }
    frame "X10" {
      (unwired) 1 items=["-----", "A", "B", "C", "D", "E", "F", "G", "H", "I", "J", "K", "L", "M", "N", "O", "P"] ("House Code")
      n521 = Greater Than 0?(x=w1401) -> (x > 0?=w1400:bool)
      n522 = Unbundle By Name(w1406) -> ("Port Name"=w1403:string, "Main"=w1404:i32, "Ch."=w1405:i32)
      n523 = call "X10control.vi"("Port Name"=w1403, "Power Request (ON)"=w1400, "House Code"=w1404, "Unit No."=w1405) -> ()  [unwired: 6 out]
      n524 = Select(t=1.0, s=w1400, f=0.0) -> (s? t:f=w1397:dbl)
    }
  }
  "Output" <- w8
  "Scan comment" <- w5
